vi "Strategy 5_Autotuning PID_With GUI Modified for Testing_Corrupted.vi"() -> ()   [LabVIEW 2018]
doc: "This example demonstrates how to use the PID Design function to obtain PID parameters based on measured process."
uses:
  <vilib>/DAQmx/write.llb/DAQmx Write (Digital 1D Bool 1Chan 1Samp).vi
  <vilib>/DAQmx/read.llb/DAQmx Read (Analog 1D DBL NChan 1Samp).vi
  <vilib>/Instr/_visa.llb/VISA Configure Serial Port (Instr).vi
  <vilib>/DAQmx/create/channels.llb/DAQmx Create Channel (DO-Digital Output).vi
  <vilib>/DAQmx/miscellaneous.llb/DAQmx Fill In Error Info.vi
  <vilib>/addons/control/pid/pid.llb/PID Advanced (DBL).vi
  <vilib>/addons/control/pid/autopid.llb/PID Autotuning Design (Ziegler-Nichols).vi
  <vilib>/addons/control/pid/autopid.llb/PID Autotuning Design (Cohen-Coon).vi
  <vilib>/addons/control/pid/autopid.llb/PID Autotuning Design (Chien-Hrones-Reswick).vi
  <vilib>/addons/control/pid/autopid.llb/PID Autotuning Design (Internal Model Control).vi
  <vilib>/addons/control/pid/NI_PID_autopid.lvlib
  <vilib>/addons/control/pid/NI_PID_pid.lvlib
  <vilib>/ptbypt/NI_PtbyPt.lvlib
panel:
  out "Tracker 4 - X,Y,Z":cluster{"x":sgl, "y":sgl, "z":sgl}(graph)
  out "Tracker 3 - X,Y,Z":cluster{"x":sgl, "y":sgl, "z":sgl}(graph)
  out "Tracker 2 - X,Y,Z":cluster{"x":sgl, "y":sgl, "z":sgl}(graph)
  out "Tracker 1 - X,Y,Z":cluster{"x":sgl, "y":sgl, "z":sgl}(graph)
  in  "Set Point 1,5":dbl
  out "Real time Data 1,5":dbl[][](graph)
  in  "Set Point 3,4":dbl
  out "Real time Data 3,4":dbl[][](graph)
  in  "Set Point 2":dbl
  out "Real time Data 2":dbl[][](graph)
  in  "Set Point 7":dbl
  out "Real time Data 7":dbl[][](graph)
  in  "Set Point  6,8,9,10":dbl
  out "Real time Data 6,8,9,10":dbl[][](graph)
  in  "Set Point 11,12":dbl
  out "Real time Data -11,12":dbl[][](graph)
  out "error out":errorcluster {"code" format="%.0x"}
  in  "XYZAER":T1(array[cluster]) {"r" format="%1_6f"; "e" format="%1_6f"; "a" format="%1_6f"; "z" format="%1_6f"; "y" format="%1_6f"; "x" format="%1_6f"}
  out "Start Time Text":string
  out "Stop Time Text":string
  out "Elapsed Time Text":string
  out "HostFrameCount":u32
  out "Loop Iter":i32
  out "PnoData":bool
  in  "stop":bool
  out "?":bool
  in  "Muscle Control":T2(tab)=enum."M-11,12"
  out "Tuned PID gains 12":T3={"proportional gain (Kc)"=1.9838195929127882, "integral time (Ti, min)"=0.01995856284686879, "derivative time (Td, min)"=0.0} {"derivative time (Td, min)" format="%#.6g"; "integral time (Ti, min)" format="%#.6g"; "proportional gain (Kc)" format="%#.6g"}
  in  "Accept gain 12":bool
  in  "Control 12":T4(tab)
  in  "Ziegler-Nichols speed 12":u16(ring) items=["Fast", "Normal", "Slow"]
  in  "Tuning specifications 12":u16(ring) items=["Regulator - 0 %", "Regulator -  20%", "Servo - 0%", "Servo - 20%"]
  in  "Multiplicative factor 12":dbl(slide)=1.0 scale=0.01..100.0
  in  "Type of controller 12":u16(ring)=2 items=["P", "PI", "PID"]
  in  "Stop 12":bool
  in  "PID Gains 12":T3={"proportional gain (Kc)"=0.1625, "integral time (Ti, min)"=1.25, "derivative time (Td, min)"=0.0} {"derivative time (Td, min)" format="%#.6g"; "integral time (Ti, min)" format="%#.6g"; "proportional gain (Kc)" format="%#.6g"}
  in  "Autotune 12":bool
  in  "Reinitialize 12":bool
  in  "Excitation 12":dbl=0.5 format="%.2f"
  in  "Automatic 12":bool=TRUE
  in  "MV: 12":dbl(slide)=20.39115328927357 scale=-100.0..100.0
  out "PWM Output 12":bool
  in  "Median sample length 21":i32=100
  in  "INLET 1,5 ON/OFF 3":bool=TRUE
  out "Tuned PID gains 9":T3={"proportional gain (Kc)"=1.9838195929127882, "integral time (Ti, min)"=0.01995856284686879, "derivative time (Td, min)"=0.0} {"derivative time (Td, min)" format="%#.6g"; "integral time (Ti, min)" format="%#.6g"; "proportional gain (Kc)" format="%#.6g"}
  in  "Accept gain 9":bool
  in  "Type of controller 9":u16(ring)=2 items=["P", "PI", "PID"]
  in  "Excitation 9":dbl=0.5 format="%.2f"
  in  "Control 9":T4(tab)
  in  "Ziegler-Nichols speed 9":u16(ring) items=["Fast", "Normal", "Slow"]
  in  "Tuning specifications 9":u16(ring) items=["Regulator - 0 %", "Regulator -  20%", "Servo - 0%", "Servo - 20%"]
  in  "Multiplicative factor 9":dbl(slide)=1.0 scale=0.01..100.0
  in  "Stop 9":bool
  in  "PID Gains 9":T3={"proportional gain (Kc)"=0.1625, "integral time (Ti, min)"=1.25, "derivative time (Td, min)"=0.0} {"derivative time (Td, min)" format="%#.6g"; "integral time (Ti, min)" format="%#.6g"; "proportional gain (Kc)" format="%#.6g"}
  in  "Autotune 9":bool
  in  "Reinitialize 9":bool
  in  "Automatic 9":bool=TRUE
  in  "MV: 9":dbl(slide)=20.39115328927357 scale=-100.0..100.0
  out "PWM Output 9":bool
  in  "Median sample length 18":i32=100
  in  "INLET 3,4 ON/OFF 2":bool=TRUE
  out "Tuned PID gains 8":T3={"proportional gain (Kc)"=1.9838195929127882, "integral time (Ti, min)"=0.01995856284686879, "derivative time (Td, min)"=0.0} {"derivative time (Td, min)" format="%#.6g"; "integral time (Ti, min)" format="%#.6g"; "proportional gain (Kc)" format="%#.6g"}
  in  "Accept gain 8":bool
  in  "Control 8":T4(tab)
  in  "Ziegler-Nichols speed 8":u16(ring) items=["Fast", "Normal", "Slow"]
  in  "Tuning specifications 8":u16(ring) items=["Regulator - 0 %", "Regulator -  20%", "Servo - 0%", "Servo - 20%"]
  in  "Multiplicative factor 8":dbl(slide)=1.0 scale=0.01..100.0
  in  "Type of controller 8":u16(ring)=2 items=["P", "PI", "PID"]
  in  "Stop 8":bool
  in  "PID Gains 8":T3={"proportional gain (Kc)"=0.1625, "integral time (Ti, min)"=1.25, "derivative time (Td, min)"=0.0} {"derivative time (Td, min)" format="%#.6g"; "integral time (Ti, min)" format="%#.6g"; "proportional gain (Kc)" format="%#.6g"}
  in  "Autotune 8":bool
  in  "Reinitialize 8":bool
  in  "Excitation 8":dbl=0.5 format="%.2f"
  in  "Automatic 8":bool=TRUE
  in  "MV: 8":dbl(slide)=20.39115328927357 scale=-100.0..100.0
  out "PWM Output 8":bool
  in  "Median sample length 17":i32=100
  in  "INLET 2 ON/OFF 2":bool=TRUE
  out "Tuned PID gains 7":T3={"proportional gain (Kc)"=1.9838195929127882, "integral time (Ti, min)"=0.01995856284686879, "derivative time (Td, min)"=0.0} {"derivative time (Td, min)" format="%#.6g"; "integral time (Ti, min)" format="%#.6g"; "proportional gain (Kc)" format="%#.6g"}
  in  "Accept gain 7":bool
  in  "Control 7":T4(tab)
  in  "Ziegler-Nichols speed 7":u16(ring) items=["Fast", "Normal", "Slow"]
  in  "Tuning specifications 7":u16(ring) items=["Regulator - 0 %", "Regulator -  20%", "Servo - 0%", "Servo - 20%"]
  in  "Multiplicative factor 7":dbl(slide)=1.0 scale=0.01..100.0
  in  "Type of controller 7":u16(ring)=2 items=["P", "PI", "PID"]
  in  "Stop 7":bool
  in  "PID Gains 7":T3={"proportional gain (Kc)"=0.1625, "integral time (Ti, min)"=1.25, "derivative time (Td, min)"=0.0} {"derivative time (Td, min)" format="%#.6g"; "integral time (Ti, min)" format="%#.6g"; "proportional gain (Kc)" format="%#.6g"}
  in  "Autotune 7":bool
  in  "Reinitialize 7":bool
  in  "Excitation 7":dbl=0.5 format="%.2f"
  in  "Automatic 7":bool=TRUE
  in  "MV: 7":dbl(slide)=20.39115328927357 scale=-100.0..100.0
  out "PWM Output 7":bool
  in  "Median sample length 16":i32=100
  in  "INLET 7 ON/OFF 2":bool=TRUE
  out "Tuned PID gains 6":T3={"proportional gain (Kc)"=1.9838195929127882, "integral time (Ti, min)"=0.01995856284686879, "derivative time (Td, min)"=0.0} {"derivative time (Td, min)" format="%#.6g"; "integral time (Ti, min)" format="%#.6g"; "proportional gain (Kc)" format="%#.6g"}
  in  "Accept gain 6":bool
  in  "Control 6":T4(tab)
  in  "Ziegler-Nichols speed 6":u16(ring) items=["Fast", "Normal", "Slow"]
  in  "Tuning specifications 6":u16(ring) items=["Regulator - 0 %", "Regulator -  20%", "Servo - 0%", "Servo - 20%"]
  in  "Multiplicative factor 6":dbl(slide)=1.0 scale=0.01..100.0
  in  "Type of controller 6":u16(ring)=2 items=["P", "PI", "PID"]
  in  "Stop 6":bool
  in  "PID Gains 6":T3={"proportional gain (Kc)"=0.1625, "integral time (Ti, min)"=1.25, "derivative time (Td, min)"=0.0} {"derivative time (Td, min)" format="%#.6g"; "integral time (Ti, min)" format="%#.6g"; "proportional gain (Kc)" format="%#.6g"}
  in  "Autotune 6":bool
  in  "Reinitialize 6":bool
  in  "Excitation 6":dbl=0.5 format="%.2f"
  in  "Automatic 6":bool=TRUE
  in  "MV: 6":dbl(slide)=20.39115328927357 scale=-100.0..100.0
  out "PWM Output 6":bool
  in  "Median sample length 15":i32=100
  in  "INLET 6 ON/OFF 2":bool=TRUE
  in  "INLET":bool=TRUE
  out "PWM Output":bool
  in  "MV:":dbl(slide)=20.39115328927357 scale=-100.0..100.0
  in  "Median sample length":i32=100
  in  "Excitation":dbl=0.5 format="%.2f"
  in  "Type of controller":u16(ring)=2 items=["P", "PI", "PID"]
  in  "Control":T4(tab)
  in  "Ziegler-Nichols speed":u16(ring) items=["Fast", "Normal", "Slow"]
  in  "Tuning specifications":u16(ring) items=["Regulator - 0 %", "Regulator -  20%", "Servo - 0%", "Servo - 20%"]
  in  "Multiplicative factor":dbl(slide)=1.0 scale=0.01..100.0
  in  "Automatic":bool=TRUE
  in  "Reinitialize":bool
  in  "Accept gain":bool
  out "Tuned PID gains":T3={"proportional gain (Kc)"=1.9838195929127882, "integral time (Ti, min)"=0.01995856284686879, "derivative time (Td, min)"=0.0} {"derivative time (Td, min)" format="%#.6g"; "integral time (Ti, min)" format="%#.6g"; "proportional gain (Kc)" format="%#.6g"}
  in  "Autotune":bool
  in  "PID Gains":T3={"proportional gain (Kc)"=0.1625, "integral time (Ti, min)"=1.25, "derivative time (Td, min)"=0.0} {"derivative time (Td, min)" format="%#.6g"; "integral time (Ti, min)" format="%#.6g"; "proportional gain (Kc)" format="%#.6g"}
  in  "Stop":bool
  in  "M-11,12":i32=5
  in  "M-6,8,9,10":i32=5
  in  "M-7":i32=5
  in  "M-2":i32=5
  in  "M-3,4":i32=5
  in  "M-1,5":i32=5
  out "Stimulus operating point 12":dbl=20.314221540357543
  out "Response operating point 12":dbl=51.08345461694337
  out "Identified Plant Parameters 12":T5={"Plant Gain (K)"=1.7609511324977591, "Time Constant (T)"=1.9621978490901302, "Dead Time (L)"=0.22467425343567116}
  out "Control Output 12":dbl[](graph)
  out "Measurement 12":dbl[](graph)
  out "Stimulus operating point 9":dbl=20.314221540357543
  out "Response operating point 9":dbl=51.08345461694337
  out "Identified Plant Parameters 9":T5={"Plant Gain (K)"=1.7609511324977591, "Time Constant (T)"=1.9621978490901302, "Dead Time (L)"=0.22467425343567116}
  out "Control Output 9":dbl[](graph)
  out "Measurement 9":dbl[](graph)
  out "Identified Plant Parameters":T5={"Plant Gain (K)"=1.7609511324977591, "Time Constant (T)"=1.9621978490901302, "Dead Time (L)"=0.22467425343567116}
  out "Control Output":dbl[](graph)
  out "Measurement":dbl[](graph)
  out "Stimulus operating point":dbl=20.314221540357543
  out "Response operating point":dbl=51.08345461694337
  out "Stimulus operating point 6":dbl=20.314221540357543
  out "Response operating point 6":dbl=51.08345461694337
  out "Identified Plant Parameters 6":T5={"Plant Gain (K)"=1.7609511324977591, "Time Constant (T)"=1.9621978490901302, "Dead Time (L)"=0.22467425343567116}
  out "Control Output 6":dbl[](graph)
  out "Measurement 6":dbl[](graph)
  out "Stimulus operating point 7":dbl=20.314221540357543
  out "Response operating point 7":dbl=51.08345461694337
  out "Identified Plant Parameters 7":T5={"Plant Gain (K)"=1.7609511324977591, "Time Constant (T)"=1.9621978490901302, "Dead Time (L)"=0.22467425343567116}
  out "Control Output 7":dbl[](graph)
  out "Measurement 7":dbl[](graph)
  out "Stimulus operating point 8":dbl=20.314221540357543
  out "Response operating point 8":dbl=51.08345461694337
  out "Identified Plant Parameters 8":T5={"Plant Gain (K)"=1.7609511324977591, "Time Constant (T)"=1.9621978490901302, "Dead Time (L)"=0.22467425343567116}
  out "Control Output 8":dbl[](graph)
  out "Measurement 8":dbl[](graph)
  out "Connected":bool
  out "Running":bool
  out "Position Sensor Data":cluster{dbl, "x":sgl}[](graph)
  out "Sensor Raw Value 2":i32
  in  "COM Port-Sensor 2":refnum<visa-resource-name>="COM5"
  in  "upper/lower infle":enum32{"Page 1", "Page 2"}(tab)
  out "Force in Kilograms":dbl(graph)
  out "Force in Newtons":dbl(graph)
  in  "lower/upper infle":enum32{"Page 1", "Page 2"}(tab)
  out "Force in Newtons 2":dbl(graph)
  out "Force in Kilograms 2":dbl(graph)
  in  "COM Port-Sensor 1":refnum<visa-resource-name>="COM4"
  out "Sensor Raw Value":i32
  in  "Tab Control":T6(tab)
  in  "Instructions":string="Overview: This example demonstrates how to use the PID Autotuning Design to obtain PID parameters based on setpoint and process variable collected in another loop.\nInstructions:\n1. Run the VI and wait until the process variable (PV) reaches near setpoint (SP).\n2.  In the PID Autotuning Design section, select the type of algorithm, type of controller and excitation amplitude for the 'open loop step response'. Then, click Autotune to start the process. Select the Identified Plant Parameter tab and see the results from the identification.\n3.  When the tuned PID gains do not change anymore, the identification is done and you have the option to accept by clicking Accept gain, which will transfer the new gain to PID Gains.\n4. Click the Autotune button again to go back to the automatic control state. You can try different options and repeat this process.\n5. Click Stop to stop the VI.\n"
  # "Pressure Alarm"
  # "Force Sensor Data"
  # "Position Sensor Data"
  # "PID Controller"
  # "PID Autotuning Design"
  # "No additional parameters"
  # "PID Controller"
  # "PID Autotuning Design"
  # "No additional parameters"
  # "PID Controller"
  # "PID Autotuning Design"
  # "No additional parameters"
  # "PID Controller"
  # "PID Autotuning Design"
  # "No additional parameters"
  # "PID Controller"
  # "PID Autotuning Design"
  # "No additional parameters"
  # "Muscle Control"
  # "PID Controller"
  # "PID Autotuning Design"
  # "No additional parameters"
  # "Pressure Cut Off to trigger the alarm"
  # "M-11,12"
  # "M-3,4"
  # "M-1,5"
  # "M-6,8,9,10"
  # "M-7"
  # "M-2"
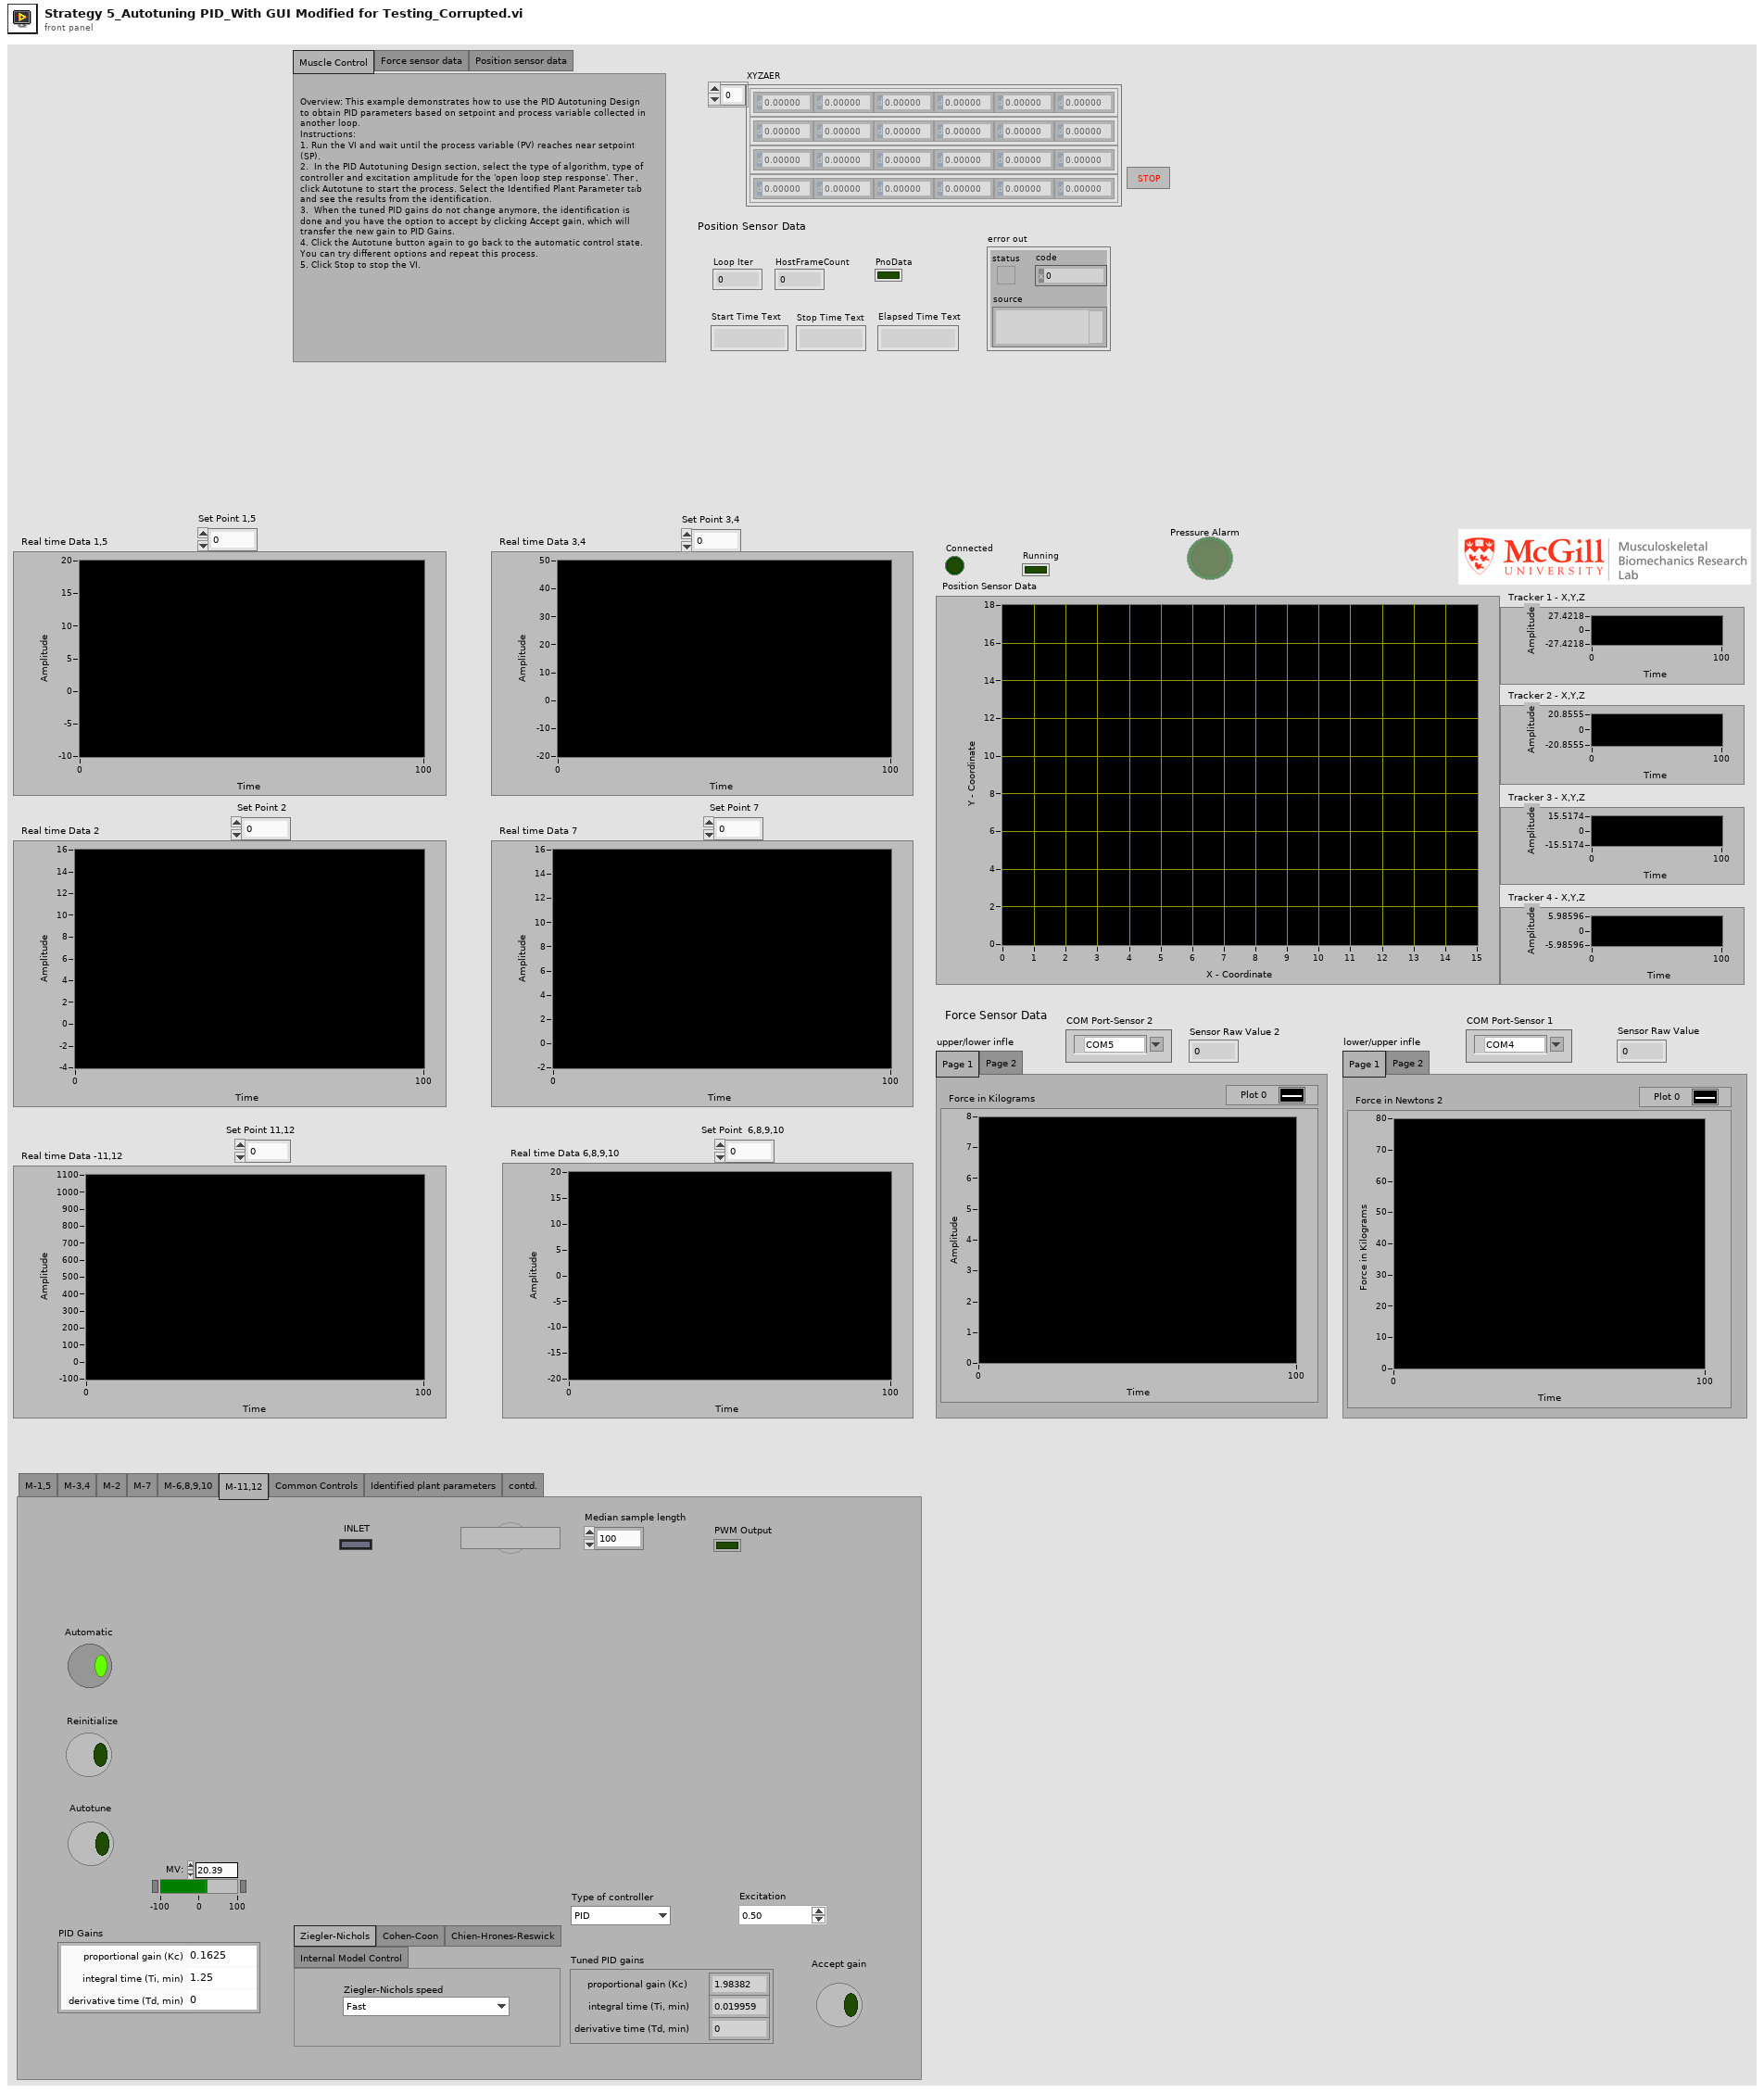
[diagram p1: front panel]
types:
  T1 = cluster{"x":sgl, "y":sgl, "z":sgl, "a":sgl, "e":sgl, "r":sgl}[]
  T2 = enum32{"M-1,5", "M-3,4", "M-2", "M-7", "M-6,8,9,10", "M-11,12", "Common Controls", "Identified plant parameters", "contd."}
  T3 = cluster{"proportional gain (Kc)":dbl, "integral time (Ti, min)":dbl, "derivative time (Td, min)":dbl}
  T4 = enum32{"Ziegler-Nichols", "Cohen-Coon", "Chien-Hrones-Reswick", "Internal Model Control"}
  T5 = cluster{"Plant Gain (K)":dbl, "Time Constant (T)":dbl, "Dead Time (L)":dbl}
  T6 = enum32{"Muscle Control", "Force sensor data", "Position sensor data"}
  T7 = cluster{"static gain":dbl, "lag (s)":dbl, "deadtime (s)":dbl, "load":dbl, "deadband":dbl, "sensor noise":dbl, "initial PV":dbl, "plant noise":dbl}
  T8 = cluster{"x":sgl, "y":sgl, "z":sgl, "a":sgl, "e":sgl, "r":sgl}
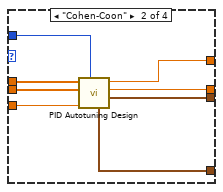
[diagram p2: hidden frame]
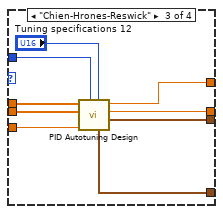
[diagram p3: hidden frame]
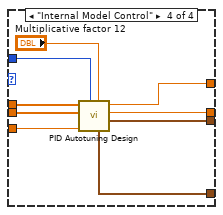
[diagram p4: hidden frame]
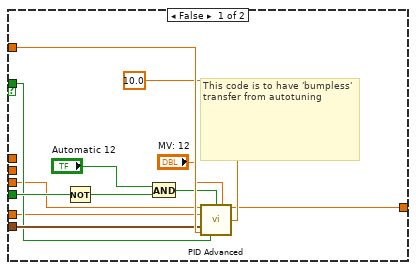
[diagram p6: hidden frame]
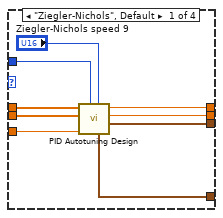
[diagram p7: hidden frame]
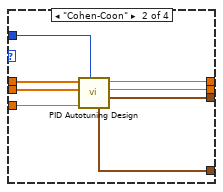
[diagram p8: hidden frame]
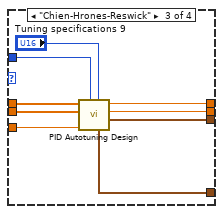
[diagram p9: hidden frame]
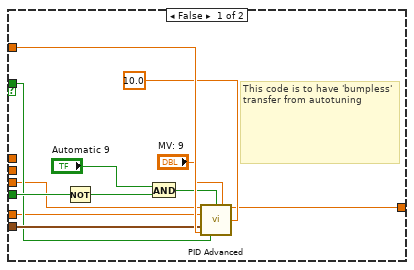
[diagram p11: hidden frame]
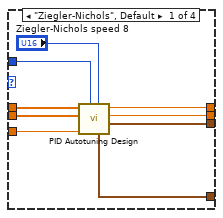
[diagram p12: hidden frame]
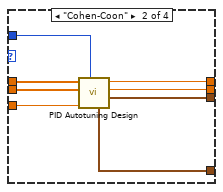
[diagram p13: hidden frame]
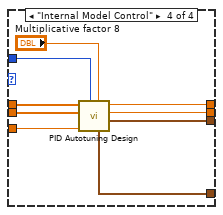
[diagram p14: hidden frame]
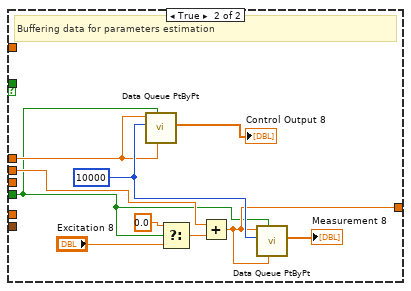
[diagram p16: hidden frame]
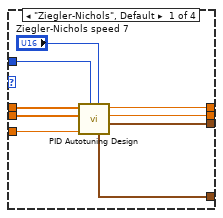
[diagram p17: hidden frame]
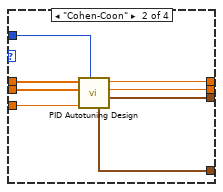
[diagram p18: hidden frame]
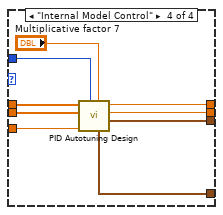
[diagram p19: hidden frame]
diagram:
  w19 = 0.0 ("output")
  w22 = FALSE ("Stop")
  w25 = 0.0 ("output")
  w28 = FALSE ("Stop")
  w31 = 0.0 ("output")
  w34 = FALSE ("Stop")
  w36 = 0.0 ("output")
  w42 = 0.0 ("output")
  w45 = FALSE ("Stop")
  w50 = 2400  # BufferFrameCount
  w83 = 0.0 ("output")
  # "Muscle-1,5 PID CONTROL LOOP (Auto Tuning)"
  # "Muscle-3,4 PID CONTROL LOOP (Auto Tuning)"
  # "Muscle-2 PID CONTROL LOOP (Auto Tuning)"
  # "Muscle-7 PID CONTROL LOOP (Auto Tuning)"
  # "Muscle-6,8,9,10 PID CONTROL LOOP (Auto Tuning)"
  # "Muscle-11,12 PID CONTROL LOOP (Auto Tuning)"
  # "FORCE SENSOR CONTROL LOOP"
  # "POSITION SENSOR CONTROL LOOP"
  # "Pressure Alarm"
  # "8. Close Tracker connection."
  # "3. Query Max num sensors supported by the tracker."
  # "4. Allocate raw buffer to hold 2400 frames of data."
  # "5. Start Continuous mode."
  # "7. Stop Continuous mode."
  # "6. Start the loop. Loop exits when Stop Button is hit."
  n1 = Obtain Queue(element data type=0.0) -> (queue out=w12:refnum<queue>)  [unwired: 4 in, 2 out]
  n2 = while {
    shift-left: 0.0 ("Plant Output") -> [w202]
    shift-right: [w197] -> _
    tunnel: w45 -> [_]
    shift-right: [w183] -> _
    shift-left: 0.01 -> [w181]
    shift-right: [w156] -> _
    shift-left: TRUE -> [w180]
    shift-right: [w158] -> _
    shift-left: w42 -> [w179]
    shift-right: [w182] -> _
    shift-left: w42 -> [w178]
    tunnel: [w153] -> w41
    tunnel: [w140] -> w2
    tunnel: w12 -> [w138]
    stop <- "Stop 6" stop-if-true
    w91 = 1 items=["one channel for each line", "one channel for all lines"] ("line grouping")
    w99 = 1 items=["one channel for each line", "one channel for all lines"] ("line grouping")
    w107 = 1 items=["one channel for each line", "one channel for all lines"] ("line grouping")
    w115 = 1 items=["one channel for each line", "one channel for all lines"] ("line grouping")
    w123 = 1 items=["one channel for each line", "one channel for all lines"] ("line grouping")
    w131 = 1 items=["one channel for each line", "one channel for all lines"] ("line grouping")
    w144 = 1 items=["one channel for each line", "one channel for all lines"] ("line grouping")
    w153 = 0.05 ("Sampling Time dt (s)")
    w161 = 1 items=["one channel for each line", "one channel for all lines"] ("line grouping")
    w169 = 0.5 ("x")
    w196 = T7 {"static gain"=2.5, "lag (s)"=2.5, "deadtime (s)"=0.01, "load"=0.0, "deadband"=0.0, "sensor noise"=0.0, "initial PV"=30.0, "plant noise"=0.0}  # Process parameters
    w198 = FALSE  # Integrator ?
    # "Inlet 11"
    # "Exhaust 10"
    # "Inlet 11"
    # "Exhaust 9"
    # "Inlet 11"
    # "Exhaust 8"
    # "C."
    # "Inlet 11"
    # "Exhaust 6"
    # "B."
    # "A."
    # "A.Output to PWM Logic \nB. Simulated Plant\nC. Draw Chart"
    # "Main PID Loop Control"
    n3 = Dequeue Element(queue=w138) -> (element=w139:dbl)  [unwired: 2 in, 3 out]
    n4 = Multiply(x=w153, y=1000.0) -> (x*y=w195:dbl)
    n5 = Not(x="Autotune 6") -> (.not. x?=w199:bool)
    n6 = feedback #1() -> (w204:bool)  [unwired: 1 in]
    n7 = feedback-in #1("Autotune 6") -> ()
    n8 = Wait Until Next ms Multiple(millisecond multiple=w195) -> ()  [unwired: 1 out]
    n9 = Exclusive Or(1:w204, 2:"Autotune 6") -> (0:w203:bool)
    n10 = feedback #2() -> (w201:dbl)  [unwired: 1 in]
    n11 = Multiply(x=w139, y=-1000.0) -> (x*y=w185:dbl)
    n12 = call <vilib>:"Median PtByPt.vi"("sample length"="Median sample length 15", "x"=w185) -> ("median"=w184:dbl)  [unwired: 2 in, 1 out]
    n13 = Square(x=w184) -> (x^2=w192:dbl)
    n14 = Multiply(x=w184, y=16.572) -> (x*y=w188:dbl)
    n15 = Multiply(x=w192, y=-0.06) -> (x*y=w189:dbl)
    n16 = Add(x=w188, y=w189) -> (x+y=w187:dbl)
    n17 = Add(x=-1011.3, y=w187) -> (x+y=w151:dbl)
    n18 = case shown="False" "Autotune 6" {
      tunnel: w153 -> [w219 _]
      tunnel: [w208 w224] -> w158
      tunnel: w202 -> [_ w223]
      tunnel: "PID Gains 6" -> [w218 _]
      tunnel: "Reinitialize 6" -> [w215 _]
      tunnel: w203 -> [w217 w222]
      tunnel: w201 -> [_ w226]
      tunnel: w151 -> [w211 _]
      tunnel: "Set Point  6,8,9,10" -> [w210 _]
      frame False {
        # "This code is to have 'bumpless' transfer from autotuning"
        n19 = Not(x=w217) -> (.not. x?=w214:bool)
        n20 = And(x="Automatic 6", y=w214) -> (x .and. y?=w216:bool)
        n21 = call-poly <vilib>:"PID Advanced.vi"("setpoint"=w210, "auto? (T)"=w216, "manual control"="MV: 6", "process variable"=w211, "alpha"=10.0, "PID gains"=w218, "dt (s)"=w219, "reinitialize? (F)"=w215) -> ("output"=w208:dbl)  [unwired: 6 in, 1 out]
      }
      frame True {
        w229 = 10000 ("sample length")
        # "Buffering data for parameters estimation"
        n22 = call <vilib>:"Data Queue PtByPt.vi"("initial queue element"=w223, "initialize"=w222, "sample length"=w229, "input data point"=w223) -> ("Current Queue"=→"Control Output 6":dbl[])  [unwired: 3 in, 4 out]
        n23 = Select(t=0.0, s=w222, f="Excitation 6") -> (s? t:f=w227:dbl)
        n24 = Add(x=w226, y=w227) -> (x+y=w224:dbl)
        n25 = call <vilib>:"Data Queue PtByPt.vi"("initial queue element"=w224, "initialize"=w222, "sample length"=w229, "input data point"=w224) -> ("Current Queue"=→"Measurement 6":dbl[])  [unwired: 3 in, 4 out]
      }
    }
    n26 = feedback-in #2(w158, w199) -> ()
    n27 = Greater?(x=w151, y="M-6,8,9,10") -> (0:w140:bool)
    n28 = Add(x=w181, y=w169) -> (x+y=w170:dbl)
    n29 = Subtract(x=w181, y=w169) -> (x-y=w168:dbl)
    n30 = Equal?(x=w179, y=w158) -> (x = y?=w176:bool)
    n31 = Greater?(x=w158, y=w179) -> (0:w175:bool)
    n32 = Select(t=w180, s=w176, f=w175) -> (s? t:f=w156:bool)
    "PWM Output 6" <- w156
    n33 = call "Plant System.vi"("Integrator ?"=w198, "Plant Input"=w158, "dt (s)"=w153, "process parameters"=w196) -> ("Plant Output"=w197:dbl)  [unwired: 11 in]
    n34 = Increment(x="Set Point  6,8,9,10") -> (x+1=w174:dbl)
    n35 = Decrement(x="Set Point  6,8,9,10") -> (x-1=w173:dbl)
    n36 = Select(t=w170, s=w156, f=w168) -> (s? t:f=w183:dbl)
    n37 = call-poly <vilib>:"DAQmx Create Virtual Channel.vi"("lines"=tag "cDAQ1Mod1/port0/line3", "line grouping"=w115) -> ("task out"=w117:refnum<k21>, "error out"=w116:errorcluster)  [unwired: 12 in]
    n38 = call-poly <vilib>:"DAQmx Create Virtual Channel.vi"("lines"=tag "cDAQ1Mod2/port0/line3", "line grouping"=w107) -> ("task out"=w109:refnum<k21>, "error out"=w108:errorcluster)  [unwired: 12 in]
    n39 = Select(t=w174, s=w156, f=w173) -> (s? t:f=w172:dbl)
    n40 = Not(x=w156) -> (.not. x?=w155:bool)
    n41 = call-poly <vilib>:"DAQmx Create Virtual Channel.vi"("lines"=tag "cDAQ1Mod1/port0/line4", "line grouping"=w161) -> ("task out"=w163:refnum<k21>, "error out"=w162:errorcluster)  [unwired: 12 in]
    n42 = call-poly <vilib>:"DAQmx Create Virtual Channel.vi"("lines"=tag "cDAQ1Mod2/port0/line4", "line grouping"=w144) -> ("task out"=w146:refnum<k21>, "error out"=w145:errorcluster)  [unwired: 12 in]
    n43 = Build Array(w151, "Set Point  6,8,9,10", w172) -> (w171:dbl[])
    n44 = Initialize Array("INLET 6 ON/OFF 2", 1 ("dimension size")) -> (w88:bool[])
    n45 = Initialize Array(w155, 1 ("dimension size")) -> (w89:bool[])
    n46 = local write "MV: 6"(w158) -> ()
    n47 = Add(x=w178, y=w181) -> (x+y=w182:dbl)
    n48 = Build Array(w171) -> (→"Real time Data 6,8,9,10":dbl[][])
    n49 = call-poly <vilib>:"DAQmx Write.vi"("task/channels in"=w117, "auto start"=TRUE, "data"=w89, "error in"=w116) -> ("task out"=w119:refnum<k21>, "error out"=w120:errorcluster)  [unwired: 9 in, 1 out]
    n50 = call-poly <vilib>:"DAQmx Write.vi"("task/channels in"=w109, "auto start"=TRUE, "data"=w88, "error in"=w108) -> ("task out"=w111:refnum<k21>, "error out"=w112:errorcluster)  [unwired: 9 in, 1 out]
    n51 = call-poly <vilib>:"DAQmx Write.vi"("task/channels in"=w163, "auto start"=TRUE, "data"=w89, "error in"=w162) -> ("task out"=w165:refnum<k21>, "error out"=w166:errorcluster)  [unwired: 9 in, 1 out]
    n52 = call-poly <vilib>:"DAQmx Write.vi"("task/channels in"=w146, "auto start"=TRUE, "data"=w88, "error in"=w145) -> ("task out"=w148:refnum<k21>, "error out"=w149:errorcluster)  [unwired: 9 in, 1 out]
    n53 = call <vilib>:"DAQmx Clear Task.vi"("task in"=w119, "error in"=w120) -> ("error out"=w114:errorcluster)  [unwired: 13 in]
    n54 = call <vilib>:"DAQmx Clear Task.vi"("task in"=w111, "error in"=w112) -> ("error out"=w106:errorcluster)  [unwired: 13 in]
    n55 = call <vilib>:"DAQmx Clear Task.vi"("task in"=w165, "error in"=w166) -> ("error out"=w160:errorcluster)  [unwired: 13 in]
    n56 = call <vilib>:"DAQmx Clear Task.vi"("task in"=w148, "error in"=w149) -> ("error out"=w143:errorcluster)  [unwired: 13 in]
    n57 = call <vilib>:"Simple Error Handler.vi"("error in (no error)"=w114) -> ()  [unwired: 4 in, 5 out]
    n58 = call <vilib>:"Simple Error Handler.vi"("error in (no error)"=w106) -> ()  [unwired: 4 in, 5 out]
    n59 = call <vilib>:"Simple Error Handler.vi"("error in (no error)"=w160) -> ()  [unwired: 4 in, 5 out]
    n60 = call <vilib>:"Simple Error Handler.vi"("error in (no error)"=w143) -> ()  [unwired: 4 in, 5 out]
    n61 = call-poly <vilib>:"DAQmx Create Virtual Channel.vi"("lines"=tag "cDAQ1Mod8/port0/line6", "line grouping"=w99) -> ("task out"=w101:refnum<k21>, "error out"=w100:errorcluster)  [unwired: 12 in]
    n62 = call-poly <vilib>:"DAQmx Create Virtual Channel.vi"("lines"=tag "cDAQ1Mod7/port0/line5", "line grouping"=w91) -> ("task out"=w93:refnum<k21>, "error out"=w92:errorcluster)  [unwired: 12 in]
    n63 = call-poly <vilib>:"DAQmx Create Virtual Channel.vi"("lines"=tag "cDAQ1Mod8/port0/line3", "line grouping"=w131) -> ("task out"=w133:refnum<k21>, "error out"=w132:errorcluster)  [unwired: 12 in]
    n64 = call-poly <vilib>:"DAQmx Create Virtual Channel.vi"("lines"=tag "cDAQ1Mod7/port0/line2", "line grouping"=w123) -> ("task out"=w125:refnum<k21>, "error out"=w124:errorcluster)  [unwired: 12 in]
    n65 = call-poly <vilib>:"DAQmx Write.vi"("task/channels in"=w101, "auto start"=TRUE, "data"=w89, "error in"=w100) -> ("task out"=w103:refnum<k21>, "error out"=w104:errorcluster)  [unwired: 9 in, 1 out]
    n66 = call-poly <vilib>:"DAQmx Write.vi"("task/channels in"=w93, "auto start"=TRUE, "data"=w88, "error in"=w92) -> ("task out"=w95:refnum<k21>, "error out"=w96:errorcluster)  [unwired: 9 in, 1 out]
    n67 = call-poly <vilib>:"DAQmx Write.vi"("task/channels in"=w133, "auto start"=TRUE, "data"=w89, "error in"=w132) -> ("task out"=w135:refnum<k21>, "error out"=w136:errorcluster)  [unwired: 9 in, 1 out]
    n68 = call-poly <vilib>:"DAQmx Write.vi"("task/channels in"=w125, "auto start"=TRUE, "data"=w88, "error in"=w124) -> ("task out"=w127:refnum<k21>, "error out"=w128:errorcluster)  [unwired: 9 in, 1 out]
    n69 = call <vilib>:"DAQmx Clear Task.vi"("task in"=w103, "error in"=w104) -> ("error out"=w98:errorcluster)  [unwired: 13 in]
    n70 = call <vilib>:"DAQmx Clear Task.vi"("task in"=w95, "error in"=w96) -> ("error out"=w90:errorcluster)  [unwired: 13 in]
    n71 = call <vilib>:"DAQmx Clear Task.vi"("task in"=w135, "error in"=w136) -> ("error out"=w130:errorcluster)  [unwired: 13 in]
    n72 = call <vilib>:"DAQmx Clear Task.vi"("task in"=w127, "error in"=w128) -> ("error out"=w122:errorcluster)  [unwired: 13 in]
    n73 = call <vilib>:"Simple Error Handler.vi"("error in (no error)"=w98) -> ()  [unwired: 4 in, 5 out]
    n74 = call <vilib>:"Simple Error Handler.vi"("error in (no error)"=w90) -> ()  [unwired: 4 in, 5 out]
    n75 = call <vilib>:"Simple Error Handler.vi"("error in (no error)"=w130) -> ()  [unwired: 4 in, 5 out]
    n76 = call <vilib>:"Simple Error Handler.vi"("error in (no error)"=w122) -> ()  [unwired: 4 in, 5 out]
  }
  n77 = local write "Stop 6"(w45) -> ()
  n78 = while {
    tunnel: w45 -> [_]
    tunnel: w41 -> [_]
    stop <- w245 stop-if-true
    w230 = 0.05 ("Sampling Time dt (s)")
    # "If dT and deadtime have similar values, the identification could evaluate deadtime as zero and this generates proportional gain equal to Inf. This code avoid gain changes in this situations."
    # "Autotuning Loop"
    n79 = local read "Control Output 6"() -> (w247:dbl[])
    n80 = local read "Measurement 6"() -> (w246:dbl[])
    n81 = Multiply(x=w230, y=1000.0) -> (x*y=w232:dbl)
    n82 = Wait Until Next ms Multiple(millisecond multiple=w232) -> ()  [unwired: 1 out]
    n83 = case shown="\"Chien-Hrones-Reswick\"" "Control 6" {
      tunnel: w247 -> [w256 w264 w273 w282]
      tunnel: w246 -> [w255 w263 w272 w281]
      tunnel: [w254 w262 w271 w280] -> w235
      tunnel: [w253 w261 w270 w279] -> w234
      tunnel: w230 -> [w252 w260 w269 w278]
      tunnel: [w251 w259 w268 w277] -> w233
      tunnel: [w250 w258 w267 w276] -> w237
      tunnel: "Type of controller 6" -> [w249 w257 w266 w275]
      frame "Ziegler-Nichols", Default {
        n84 = call-poly <vilib>:"PID Autotuning Design.vi"("Ziegler-Nichols Speed"="Ziegler-Nichols speed 6", "Type of Controller"=w249, "dt (s)"=w252, "Response signal"=w255, "Stimulus signal"=w256) -> ("PID gains"=w250:T3, "response operating point"=w253:dbl, "stimulus operating point"=w254:dbl, "Plant Parameters"=w251:T5)  [unwired: 3 in]
      }
      frame "Cohen-Coon" {
        n85 = call-poly <vilib>:"PID Autotuning Design.vi"("Type of Controller"=w257, "dt (s)"=w260, "Response signal"=w263, "Stimulus signal"=w264) -> ("PID gains"=w258:T3, "response offset"=w261:dbl, "stimulus offset"=w262:dbl, "Plant Parameters"=w259:T5)  [unwired: 4 in]
      }
      frame "Chien-Hrones-Reswick" {
        n86 = call-poly <vilib>:"PID Autotuning Design.vi"("Tuning specifications"="Tuning specifications 6", "Type of Controller"=w266, "dt (s)"=w269, "Response signal"=w272, "Stimulus signal"=w273) -> ("PID gains"=w267:T3, "response offset"=w270:dbl, "stimulus offset"=w271:dbl, "Plant Parameters"=w268:T5)  [unwired: 3 in]
      }
      frame "Internal Model Control" {
        n87 = call-poly <vilib>:"PID Autotuning Design.vi"("Desired Time Constant (tau_c)"="Multiplicative factor 6", "Type of Controller"=w275, "dt (s)"=w278, "Response signal"=w281, "Stimulus signal"=w282) -> ("PID gains"=w276:T3, "response offset"=w279:dbl, "stimulus offset"=w280:dbl, "Plant Parameters"=w277:T5)  [unwired: 3 in]
      }
    }
    "Stimulus operating point 6" <- w235
    "Response operating point 6" <- w234
    "Identified Plant Parameters 6" <- w233
    n88 = Unbundle(w237) -> ("proportional gain (Kc)"=w240:dbl)  [unwired: 2 out]
    n89 = Equal?(x=w240, y=inf) -> (x = y?=w239:bool)
    n90 = feedback #3() -> (w238:T3)  [unwired: 1 in]
    n91 = Select(t=w238, s=w239, f=w237) -> (s? t:f=w236:T3)
    "Tuned PID gains 6" <- w236
    n92 = feedback-in #3(w236) -> ()
    n93 = case shown="True" "Accept gain 6" {
      tunnel: w236 -> [_ w283]
      frame False {
      }
      frame True {
        n94 = local write "PID Gains 6"(w283) -> ()
      }
    }
    n95 = local read "Stop 6"() -> (w245:bool)
  }
  n96 = local write "Stop"(FALSE ("Stop")) -> ()
  n97 = call-poly "VISA Configure Serial Port"("VISA resource name"="COM Port-Sensor 1") -> ("VISA resource name out"=w78:refnum<visa-resource-name>, "error out"=w77:errorcluster)  [unwired: 9 in, 4 out]
  n98 = call-poly "VISA Configure Serial Port"("VISA resource name"="COM Port-Sensor 2") -> ("VISA resource name out"=w73:refnum<visa-resource-name>, "error out"=w72:errorcluster)  [unwired: 9 in, 4 out]
  n99 = while {
    stop <- w299 stop-if-true
    w284 = 0.05 ("Sampling Time dt (s)")
    # "If dT and deadtime have similar values, the identification could evaluate deadtime as zero and this generates proportional gain equal to Inf. This code avoid gain changes in this situations."
    # "Autotuning Loop"
    n100 = local read "Control Output"() -> (w301:dbl[])
    n101 = local read "Measurement"() -> (w300:dbl[])
    n102 = Multiply(x=w284, y=1000.0) -> (x*y=w286:dbl)
    n103 = Wait Until Next ms Multiple(millisecond multiple=w286) -> ()  [unwired: 1 out]
    n104 = case shown="\"Ziegler-Nichols\", Default" "Control" {
      tunnel: w301 -> [w310 w318 w327 w336]
      tunnel: w300 -> [w309 w317 w326 w335]
      tunnel: [w308 w316 w325 w334] -> w289
      tunnel: [w307 w315 w324 w333] -> w288
      tunnel: w284 -> [w306 w314 w323 w332]
      tunnel: [w305 w313 w322 w331] -> w287
      tunnel: [w304 w312 w321 w330] -> w291
      tunnel: "Type of controller" -> [w303 w311 w320 w329]
      frame "Ziegler-Nichols", Default {
        n105 = call-poly <vilib>:"PID Autotuning Design.vi"("Ziegler-Nichols Speed"="Ziegler-Nichols speed", "Type of Controller"=w303, "dt (s)"=w306, "Response signal"=w309, "Stimulus signal"=w310) -> ("PID gains"=w304:T3, "response operating point"=w307:dbl, "stimulus operating point"=w308:dbl, "Plant Parameters"=w305:T5)  [unwired: 3 in]
      }
      frame "Cohen-Coon" {
        n106 = call-poly <vilib>:"PID Autotuning Design.vi"("Type of Controller"=w311, "dt (s)"=w314, "Response signal"=w317, "Stimulus signal"=w318) -> ("PID gains"=w312:T3, "response offset"=w315:dbl, "stimulus offset"=w316:dbl, "Plant Parameters"=w313:T5)  [unwired: 4 in]
      }
      frame "Chien-Hrones-Reswick" {
        n107 = call-poly <vilib>:"PID Autotuning Design.vi"("Tuning specifications"="Tuning specifications", "Type of Controller"=w320, "dt (s)"=w323, "Response signal"=w326, "Stimulus signal"=w327) -> ("PID gains"=w321:T3, "response offset"=w324:dbl, "stimulus offset"=w325:dbl, "Plant Parameters"=w322:T5)  [unwired: 3 in]
      }
      frame "Internal Model Control" {
        n108 = call-poly <vilib>:"PID Autotuning Design.vi"("Desired Time Constant (tau_c)"="Multiplicative factor", "Type of Controller"=w329, "dt (s)"=w332, "Response signal"=w335, "Stimulus signal"=w336) -> ("PID gains"=w330:T3, "response offset"=w333:dbl, "stimulus offset"=w334:dbl, "Plant Parameters"=w331:T5)  [unwired: 3 in]
      }
    }
    "Stimulus operating point" <- w289
    "Response operating point" <- w288
    "Identified Plant Parameters" <- w287
    n109 = Unbundle(w291) -> ("proportional gain (Kc)"=w294:dbl)  [unwired: 2 out]
    n110 = Equal?(x=w294, y=inf) -> (x = y?=w293:bool)
    n111 = feedback #4() -> (w292:T3)  [unwired: 1 in]
    n112 = Select(t=w292, s=w293, f=w291) -> (s? t:f=w290:T3)
    "Tuned PID gains" <- w290
    n113 = feedback-in #4(w290) -> ()
    n114 = case shown="True" "Accept gain" {
      tunnel: w290 -> [_ w337]
      frame False {
      }
      frame True {
        n115 = local write "PID Gains"(w337) -> ()
      }
    }
    n116 = local read "Stop"() -> (w299:bool)
  }
  n117 = while {
    shift-right: [w345] -> w79
    shift-left: w78 -> [w341]
    tunnel: w77 -> [w340]
    tunnel: [w342] -> w80
    stop <- w343 stop-if-true
    # "Serial Read Loop"
    n118 = case shown="True" TRUE {
      tunnel: [w357 w361] -> w345
      tunnel: w341 -> [w359 w361]
      tunnel: [w356 w360] -> w342
      tunnel: w340 -> [w358 w360]
      frame True {
        n119 = VISA Read(VISA resource name=w359, byte count=u32 1000, error in (no error)=w358) -> (VISA resource name out=w357:refnum<visa-resource-name>, read buffer=w354:string, error out=w356:errorcluster)  [unwired: 1 out]
        n120 = Decimal String To Number(string=w354) -> (number=w352:i32)  [unwired: 2 in, 1 out]
        "Sensor Raw Value" <- w352
        n121 = call <vilib>:"Median PtByPt.vi"("sample length"=20, "x"=w352) -> ("median"=w350:dbl)  [unwired: 2 in, 1 out]
        n122 = To Double Precision Float(number=w350) -> (double precision float=w346:dbl)
        n123 = Multiply(x=w346, y=0.0292) -> (x*y=w349:dbl)
        "Force in Kilograms 2" <- w349
        n124 = Multiply(x=w349, y=9.81) -> (x*y=→"Force in Newtons 2":dbl)
      }
      frame False {
      }
    }
    n125 = Wait (ms)(milliseconds to wait=u32 5) -> ()  [unwired: 1 out]
    n126 = Or(x=w342, y=FALSE) -> (x .or. y?=w343:bool)
  }
  n127 = while {
    shift-right: [w369] -> w47
    shift-left: w73 -> [w365]
    tunnel: w72 -> [w364]
    tunnel: [w366] -> w74
    stop <- w367 stop-if-true
    # "Serial Read Loop"
    n128 = case shown="True" TRUE {
      tunnel: [w381 w385] -> w369
      tunnel: w365 -> [w383 w385]
      tunnel: [w380 w384] -> w366
      tunnel: w364 -> [w382 w384]
      frame True {
        n129 = VISA Read(VISA resource name=w383, byte count=u32 1000, error in (no error)=w382) -> (VISA resource name out=w381:refnum<visa-resource-name>, read buffer=w378:string, error out=w380:errorcluster)  [unwired: 1 out]
        n130 = Decimal String To Number(string=w378) -> (number=w374:i32)  [unwired: 2 in, 1 out]
        "Sensor Raw Value 2" <- w374
        n131 = call <vilib>:"Median PtByPt.vi"("sample length"=20, "x"=w374) -> ("median"=w375:dbl)  [unwired: 2 in, 1 out]
        n132 = To Double Precision Float(number=w375) -> (double precision float=w371:dbl)
        n133 = Multiply(x=w371, y=0.0238) -> (x*y=w370:dbl)
        "Force in Kilograms" <- w370
        n134 = Multiply(x=w370, y=9.81) -> (x*y=→"Force in Newtons":dbl)
      }
      frame False {
      }
    }
    n135 = Or(x=w366, y=FALSE) -> (x .or. y?=w367:bool)
    n136 = Wait (ms)(milliseconds to wait=u32 5) -> ()  [unwired: 1 out]
  }
  n137 = VISA Close(VISA resource name=w79, error in (no error)=w80) -> (error out=w81:errorcluster)
  n138 = call <vilib>:"Simple Error Handler.vi"("error in (no error)"=w81) -> ()  [unwired: 1 in, 8 out]
  n139 = VISA Close(VISA resource name=w47, error in (no error)=w74) -> (error out=w75:errorcluster)
  n140 = call <vilib>:"Simple Error Handler.vi"("error in (no error)"=w75) -> ()  [unwired: 1 in, 8 out]
  n141 = stacked-sequence {
    tunnel: [_ w391] -> w54
    tunnel: [_ w390] -> w53
    frame #0 {
      w386 = 0
      w387 = FALSE
      w388 = ""
      # "Initialize Indicators"
      "Connected" <- w387
      "Start Time Text" <- w388
      "Stop Time Text" <- w388
      "Elapsed Time Text" <- w388
      "HostFrameCount" <- w386
      "Running" <- w387
      "Loop Iter" <- w386
      "PnoData" <- w387
    }
    frame #1 {
      # "Connect To Tracker"
      # "2. Initialize Tracker Connection"
      n142 = call <instrlib>:"PDI initialize.vi"() -> ("error out"=w390:errorcluster, "Connected"=w389:bool, "pDev"=w391:u32)  [unwired: 1 in, 4 out]
      n143 = local write "Connected"(w389) -> ()
    }
  }
  n144 = while {
    stop <- FALSE stop-if-true
    # "TRACKER 4"
    # "TRACKER 3"
    # "TRACKER 2"
    # "TRACKER 1"
    n145 = Index Array(array="XYZAER", index #1=0 ("index"), index #2=1 ("index"), index #3=2 ("index"), index #4=3 ("index")) -> (element #1=w424:T8, element #2=w423:T8, element #3=w422:T8, element #4=w421:T8)
    n146 = Unbundle By Name(w424) -> ("x"=w407:sgl, "y"=w406:sgl, "z"=w405:sgl)
    n147 = Unbundle By Name(w423) -> ("x"=w404:sgl, "y"=w403:sgl, "z"=w402:sgl)
    n148 = Multiply(x=w406, y=sgl -1.0) -> (x*y=w415:sgl)
    n149 = Multiply(x=w403, y=-1.0) -> (x*y=w414:dbl)
    n150 = Bundle(w414, "x"=w404) -> (w410:cluster{dbl, "x":sgl})  [unwired: 1 in]
    n151 = Bundle(w415, "x"=w407) -> (w411:cluster{sgl, "x":sgl})  [unwired: 1 in]
    n152 = Unbundle By Name(w422) -> ("x"=w401:sgl, "y"=w400:sgl, "z"=w399:sgl)
    n153 = Unbundle By Name(w421) -> ("x"=w398:sgl, "y"=w397:sgl, "z"=w396:sgl)
    n154 = Multiply(x=w400, y=-1.0) -> (x*y=w413:dbl)
    n155 = Multiply(x=w397, y=-1.0) -> (x*y=w412:dbl)
    n156 = Bundle(w413, "x"=w401) -> (w409:cluster{dbl, "x":sgl})  [unwired: 1 in]
    n157 = Bundle(w412, "x"=w398) -> (w408:cluster{dbl, "x":sgl})  [unwired: 1 in]
    n158 = Build Array(w411, w410, w409, w408) -> (→"Position Sensor Data":cluster{dbl, "x":sgl}[])
    n159 = Bundle("x"=w407, "y"=w406, "z"=w405) -> (→"Tracker 1 - X,Y,Z":cluster{"x":sgl, "y":sgl, "z":sgl})  [unwired: 1 in]
    n160 = Bundle("x"=w404, "y"=w403, "z"=w402) -> (→"Tracker 2 - X,Y,Z":cluster{"x":sgl, "y":sgl, "z":sgl})  [unwired: 1 in]
    n161 = Bundle("x"=w401, "y"=w400, "z"=w399) -> (→"Tracker 3 - X,Y,Z":cluster{"x":sgl, "y":sgl, "z":sgl})  [unwired: 1 in]
    n162 = Bundle("x"=w398, "y"=w397, "z"=w396) -> (→"Tracker 4 - X,Y,Z":cluster{"x":sgl, "y":sgl, "z":sgl})  [unwired: 1 in]
  }
  n163 = call <instrlib>:"PDI util stationcount.vi"("error in (no error)"=w53, "pDev"=w54) -> ("error out"=w52:errorcluster, "dup pDev"=w51:u32, "MaxCount"=w49:i32)  [unwired: 7 out]
  n164 = call <instrlib>:"PDI config setbuffer.vi"("error in (no error)"=w52, "Max sensors"=w49, "FrameCount"=w50, "pDev"=w51) -> ("error out"=w61:errorcluster, "dup pDev"=w62:u32)  [unwired: 6 out]
  n165 = flat-sequence {
    tunnel: w67 -> [_]
    tunnel: [w431] -> w63
    frame #0 {
      # "Get Start Time"
      n166 = Get Date/Time In Seconds() -> (seconds since 1Jan1904=w432:timestamp)
      n167 = Format Date/Time String(seconds (now)=w432) -> (date/time string=w433:string)  [unwired: 2 out]
      n168 = local write "Start Time Text"(w433) -> ()
      n169 = To Double Precision Float(number=w432) -> (double precision float=w431:dbl)
    }
  }
  n170 = call <instrlib>:"PDI action startcont.vi"("error in (no error)"=w61, "pDev"=w62) -> ("error out"=w68:errorcluster, "Running"=w60:bool, "dup pDev"=w67:u32)  [unwired: 7 out]
  n171 = control-ref of="HostFrameCount"() -> (w58:refnum<vi>)
  n172 = local write "Running"(w60) -> ()
  n173 = Obtain Queue(element data type=0.0) -> (queue out=w8:refnum<queue>)  [unwired: 4 in, 2 out]
  n174 = while {
    shift-left: 0.0 ("Plant Output") -> [w516]
    shift-right: [w511] -> _
    tunnel: w28 -> [_]
    shift-right: [w497] -> _
    shift-left: 0.01 -> [w495]
    shift-right: [w470] -> _
    shift-left: TRUE -> [w494]
    shift-right: [w472] -> _
    shift-left: w25 -> [w493]
    shift-right: [w496] -> _
    shift-left: w25 -> [w492]
    tunnel: [w467] -> w24
    tunnel: [w455] -> w16
    tunnel: w8 -> [w453]
    stop <- "Stop 9" stop-if-true
    w438 = 1 items=["one channel for each line", "one channel for all lines"] ("line grouping")
    w446 = 1 items=["one channel for each line", "one channel for all lines"] ("line grouping")
    w458 = 1 items=["one channel for each line", "one channel for all lines"] ("line grouping")
    w467 = 0.05 ("Sampling Time dt (s)")
    w475 = 1 items=["one channel for each line", "one channel for all lines"] ("line grouping")
    w483 = 0.5 ("x")
    w510 = T7 {"static gain"=2.5, "lag (s)"=2.5, "deadtime (s)"=0.01, "load"=0.0, "deadband"=0.0, "sensor noise"=0.0, "initial PV"=30.0, "plant noise"=0.0}  # Process parameters
    w512 = FALSE  # Integrator ?
    # "Inlet 11"
    # "Exhaust 3"
    # "C."
    # "Inlet 11"
    # "Exhaust 4"
    # "B."
    # "A."
    # "A.Output to PWM Logic \nB. Simulated Plant\nC. Draw Chart"
    # "Main PID Loop Control"
    n175 = Dequeue Element(queue=w453) -> (element=w454:dbl)  [unwired: 2 in, 3 out]
    n176 = Multiply(x=w467, y=1000.0) -> (x*y=w509:dbl)
    n177 = Not(x="Autotune 9") -> (.not. x?=w513:bool)
    n178 = feedback #5() -> (w518:bool)  [unwired: 1 in]
    n179 = feedback-in #5("Autotune 9") -> ()
    n180 = Wait Until Next ms Multiple(millisecond multiple=w509) -> ()  [unwired: 1 out]
    n181 = Exclusive Or(1:w518, 2:"Autotune 9") -> (0:w517:bool)
    n182 = feedback #6() -> (w515:dbl)  [unwired: 1 in]
    n183 = Multiply(x=w454, y=-1000.0) -> (x*y=w499:dbl)
    n184 = call <vilib>:"Median PtByPt.vi"("sample length"="Median sample length 18", "x"=w499) -> ("median"=w498:dbl)  [unwired: 2 in, 1 out]
    n185 = Square(x=w498) -> (x^2=w506:dbl)
    n186 = Multiply(x=w498, y=0.1121) -> (x*y=w502:dbl)
    n187 = Multiply(x=w506, y=0.0243) -> (x*y=w503:dbl)
    n188 = Add(x=w502, y=w503) -> (x+y=w501:dbl)
    n189 = Add(x=-235.77, y=w501) -> (x+y=w465:dbl)
    n190 = case shown="True" "Autotune 9" {
      tunnel: w467 -> [w533 _]
      tunnel: [w522 w538] -> w472
      tunnel: w516 -> [_ w537]
      tunnel: "PID Gains 9" -> [w532 _]
      tunnel: "Reinitialize 9" -> [w529 _]
      tunnel: w517 -> [w531 w536]
      tunnel: w515 -> [_ w540]
      tunnel: w465 -> [w525 _]
      tunnel: "Set Point 3,4" -> [w524 _]
      frame False {
        # "This code is to have 'bumpless' transfer from autotuning"
        n191 = Not(x=w531) -> (.not. x?=w528:bool)
        n192 = And(x="Automatic 9", y=w528) -> (x .and. y?=w530:bool)
        n193 = call-poly <vilib>:"PID Advanced.vi"("setpoint"=w524, "auto? (T)"=w530, "manual control"="MV: 9", "process variable"=w525, "alpha"=10.0, "PID gains"=w532, "dt (s)"=w533, "reinitialize? (F)"=w529) -> ("output"=w522:dbl)  [unwired: 6 in, 1 out]
      }
      frame True {
        w543 = 10000 ("sample length")
        # "Buffering data for parameters estimation"
        n194 = call <vilib>:"Data Queue PtByPt.vi"("initial queue element"=w537, "initialize"=w536, "sample length"=w543, "input data point"=w537) -> ("Current Queue"=→"Control Output 9":dbl[])  [unwired: 3 in, 4 out]
        n195 = Select(t=0.0, s=w536, f="Excitation 9") -> (s? t:f=w541:dbl)
        n196 = Add(x=w540, y=w541) -> (x+y=w538:dbl)
        n197 = call <vilib>:"Data Queue PtByPt.vi"("initial queue element"=w538, "initialize"=w536, "sample length"=w543, "input data point"=w538) -> ("Current Queue"=→"Measurement 9":dbl[])  [unwired: 3 in, 4 out]
      }
    }
    n198 = feedback-in #6(w472, w513) -> ()
    n199 = Greater?(x=w465, y="M-3,4") -> (0:w455:bool)
    n200 = Add(x=w495, y=w483) -> (x+y=w484:dbl)
    n201 = Subtract(x=w495, y=w483) -> (x-y=w482:dbl)
    n202 = Equal?(x=w493, y=w472) -> (x = y?=w490:bool)
    n203 = Greater?(x=w472, y=w493) -> (0:w489:bool)
    n204 = Select(t=w494, s=w490, f=w489) -> (s? t:f=w470:bool)
    "PWM Output 9" <- w470
    n205 = call "Plant System.vi"("Integrator ?"=w512, "Plant Input"=w472, "dt (s)"=w467, "process parameters"=w510) -> ("Plant Output"=w511:dbl)  [unwired: 11 in]
    n206 = Increment(x="Set Point 3,4") -> (x+1=w488:dbl)
    n207 = Decrement(x="Set Point 3,4") -> (x-1=w487:dbl)
    n208 = Select(t=w484, s=w470, f=w482) -> (s? t:f=w497:dbl)
    n209 = Select(t=w488, s=w470, f=w487) -> (s? t:f=w486:dbl)
    n210 = Not(x=w470) -> (.not. x?=w469:bool)
    n211 = call-poly <vilib>:"DAQmx Create Virtual Channel.vi"("lines"=tag "cDAQ1Mod8/port0/line5", "line grouping"=w475) -> ("task out"=w477:refnum<k21>, "error out"=w476:errorcluster)  [unwired: 12 in]
    n212 = call-poly <vilib>:"DAQmx Create Virtual Channel.vi"("lines"=tag "cDAQ1Mod7/port0/line4", "line grouping"=w458) -> ("task out"=w460:refnum<k21>, "error out"=w459:errorcluster)  [unwired: 12 in]
    n213 = Build Array(w465, "Set Point 3,4", w486) -> (w485:dbl[])
    n214 = Initialize Array("INLET 3,4 ON/OFF 2", 1 ("dimension size")) -> (w434:bool[])
    n215 = Initialize Array(w469, 1 ("dimension size")) -> (w436:bool[])
    n216 = local write "MV: 9"(w472) -> ()
    n217 = Add(x=w492, y=w495) -> (x+y=w496:dbl)
    n218 = Build Array(w485) -> (→"Real time Data 3,4":dbl[][])
    n219 = call-poly <vilib>:"DAQmx Write.vi"("task/channels in"=w477, "auto start"=TRUE, "data"=w436, "error in"=w476) -> ("task out"=w479:refnum<k21>, "error out"=w480:errorcluster)  [unwired: 9 in, 1 out]
    n220 = call-poly <vilib>:"DAQmx Write.vi"("task/channels in"=w460, "auto start"=TRUE, "data"=w434, "error in"=w459) -> ("task out"=w462:refnum<k21>, "error out"=w463:errorcluster)  [unwired: 9 in, 1 out]
    n221 = call <vilib>:"DAQmx Clear Task.vi"("task in"=w479, "error in"=w480) -> ("error out"=w474:errorcluster)  [unwired: 13 in]
    n222 = call <vilib>:"DAQmx Clear Task.vi"("task in"=w462, "error in"=w463) -> ("error out"=w457:errorcluster)  [unwired: 13 in]
    n223 = call <vilib>:"Simple Error Handler.vi"("error in (no error)"=w474) -> ()  [unwired: 4 in, 5 out]
    n224 = call <vilib>:"Simple Error Handler.vi"("error in (no error)"=w457) -> ()  [unwired: 4 in, 5 out]
    n225 = call-poly <vilib>:"DAQmx Create Virtual Channel.vi"("lines"=tag "cDAQ1Mod8/port0/line7", "line grouping"=w446) -> ("task out"=w448:refnum<k21>, "error out"=w447:errorcluster)  [unwired: 12 in]
    n226 = call-poly <vilib>:"DAQmx Create Virtual Channel.vi"("lines"=tag "cDAQ1Mod7/port0/line6", "line grouping"=w438) -> ("task out"=w440:refnum<k21>, "error out"=w439:errorcluster)  [unwired: 12 in]
    n227 = call-poly <vilib>:"DAQmx Write.vi"("task/channels in"=w448, "auto start"=TRUE, "data"=w436, "error in"=w447) -> ("task out"=w450:refnum<k21>, "error out"=w451:errorcluster)  [unwired: 9 in, 1 out]
    n228 = call-poly <vilib>:"DAQmx Write.vi"("task/channels in"=w440, "auto start"=TRUE, "data"=w434, "error in"=w439) -> ("task out"=w442:refnum<k21>, "error out"=w443:errorcluster)  [unwired: 9 in, 1 out]
    n229 = call <vilib>:"DAQmx Clear Task.vi"("task in"=w450, "error in"=w451) -> ("error out"=w445:errorcluster)  [unwired: 13 in]
    n230 = call <vilib>:"DAQmx Clear Task.vi"("task in"=w442, "error in"=w443) -> ("error out"=w437:errorcluster)  [unwired: 13 in]
    n231 = call <vilib>:"Simple Error Handler.vi"("error in (no error)"=w445) -> ()  [unwired: 4 in, 5 out]
    n232 = call <vilib>:"Simple Error Handler.vi"("error in (no error)"=w437) -> ()  [unwired: 4 in, 5 out]
  }
  n233 = control-ref of="stop"() -> (w66:refnum<vi>)
  n234 = control-ref of="XYZAER"() -> (w57:refnum<vi>)
  n235 = Obtain Queue(element data type=0.0) -> (queue out=w5:refnum<queue>)  [unwired: 4 in, 2 out]
  n236 = while {
    shift-left: 0.0 ("Plant Output") -> [w610]
    shift-right: [w605] -> _
    tunnel: w34 -> [_]
    shift-right: [w591] -> _
    shift-left: 0.01 -> [w589]
    shift-right: [w563] -> _
    shift-left: TRUE -> [w588]
    shift-right: [w565] -> _
    shift-left: w31 -> [w587]
    shift-right: [w590] -> _
    shift-left: w31 -> [w586]
    tunnel: [w560] -> w30
    tunnel: [w546] -> w15
    tunnel: w5 -> [w544]
    stop <- "Stop 8" stop-if-true
    w551 = 1 items=["one channel for each line", "one channel for all lines"] ("line grouping")
    w560 = 0.05 ("Sampling Time dt (s)")
    w569 = 1 items=["one channel for each line", "one channel for all lines"] ("line grouping")
    w577 = 0.5 ("x")
    w604 = T7 {"static gain"=2.5, "lag (s)"=2.5, "deadtime (s)"=0.01, "load"=0.0, "deadband"=0.0, "sensor noise"=0.0, "initial PV"=30.0, "plant noise"=0.0}  # Process parameters
    w606 = FALSE  # Integrator ?
    # "C."
    # "Inlet 11"
    # "Exhaust 2"
    # "B."
    # "A."
    # "A.Output to PWM Logic \nB. Simulated Plant\nC. Draw Chart"
    # "Main PID Loop Control"
    n237 = Dequeue Element(queue=w544) -> (element=w545:dbl)  [unwired: 2 in, 3 out]
    n238 = Multiply(x=w560, y=1000.0) -> (x*y=w603:dbl)
    n239 = Not(x="Autotune 8") -> (.not. x?=w607:bool)
    n240 = feedback #7() -> (w612:bool)  [unwired: 1 in]
    n241 = feedback-in #7("Autotune 8") -> ()
    n242 = Wait Until Next ms Multiple(millisecond multiple=w603) -> ()  [unwired: 1 out]
    n243 = Exclusive Or(1:w612, 2:"Autotune 8") -> (0:w611:bool)
    n244 = feedback #8() -> (w609:dbl)  [unwired: 1 in]
    n245 = Multiply(x=w545, y=-1000.0) -> (x*y=w593:dbl)
    n246 = call <vilib>:"Median PtByPt.vi"("sample length"="Median sample length 17", "x"=w593) -> ("median"=w592:dbl)  [unwired: 2 in, 1 out]
    n247 = Square(x=w592) -> (x^2=w600:dbl)
    n248 = Multiply(x=w592, y=-7.5945) -> (x*y=w596:dbl)
    n249 = Multiply(x=w600, y=0.0612) -> (x*y=w597:dbl)
    n250 = Add(x=w596, y=w597) -> (x+y=w595:dbl)
    n251 = Add(x=143.72, y=w595) -> (x+y=w558:dbl)
    n252 = case shown="False" "Autotune 8" {
      tunnel: w560 -> [w627 _]
      tunnel: [w616 w632] -> w565
      tunnel: w610 -> [_ w631]
      tunnel: "PID Gains 8" -> [w626 _]
      tunnel: "Reinitialize 8" -> [w623 _]
      tunnel: w611 -> [w625 w630]
      tunnel: w609 -> [_ w634]
      tunnel: w558 -> [w619 _]
      tunnel: "Set Point 2" -> [w618 _]
      frame False {
        # "This code is to have 'bumpless' transfer from autotuning"
        n253 = Not(x=w625) -> (.not. x?=w622:bool)
        n254 = And(x="Automatic 8", y=w622) -> (x .and. y?=w624:bool)
        n255 = call-poly <vilib>:"PID Advanced.vi"("setpoint"=w618, "auto? (T)"=w624, "manual control"="MV: 8", "process variable"=w619, "alpha"=10.0, "PID gains"=w626, "dt (s)"=w627, "reinitialize? (F)"=w623) -> ("output"=w616:dbl)  [unwired: 6 in, 1 out]
      }
      frame True {
        w637 = 10000 ("sample length")
        # "Buffering data for parameters estimation"
        n256 = call <vilib>:"Data Queue PtByPt.vi"("initial queue element"=w631, "initialize"=w630, "sample length"=w637, "input data point"=w631) -> ("Current Queue"=→"Control Output 8":dbl[])  [unwired: 3 in, 4 out]
        n257 = Select(t=0.0, s=w630, f="Excitation 8") -> (s? t:f=w635:dbl)
        n258 = Add(x=w634, y=w635) -> (x+y=w632:dbl)
        n259 = call <vilib>:"Data Queue PtByPt.vi"("initial queue element"=w632, "initialize"=w630, "sample length"=w637, "input data point"=w632) -> ("Current Queue"=→"Measurement 8":dbl[])  [unwired: 3 in, 4 out]
      }
    }
    n260 = feedback-in #8(w565, w607) -> ()
    n261 = Greater?(x=w558, y="M-2") -> (0:w546:bool)
    n262 = Add(x=w589, y=w577) -> (x+y=w578:dbl)
    n263 = Subtract(x=w589, y=w577) -> (x-y=w576:dbl)
    n264 = Equal?(x=w587, y=w565) -> (x = y?=w584:bool)
    n265 = Greater?(x=w565, y=w587) -> (0:w583:bool)
    n266 = Select(t=w588, s=w584, f=w583) -> (s? t:f=w563:bool)
    "PWM Output 8" <- w563
    n267 = call "Plant System.vi"("Integrator ?"=w606, "Plant Input"=w565, "dt (s)"=w560, "process parameters"=w604) -> ("Plant Output"=w605:dbl)  [unwired: 11 in]
    n268 = Increment(x="Set Point 2") -> (x+1=w582:dbl)
    n269 = Decrement(x="Set Point 2") -> (x-1=w581:dbl)
    n270 = Select(t=w578, s=w563, f=w576) -> (s? t:f=w591:dbl)
    n271 = Select(t=w582, s=w563, f=w581) -> (s? t:f=w580:dbl)
    n272 = Not(x=w563) -> (.not. x?=w562:bool)
    n273 = call-poly <vilib>:"DAQmx Create Virtual Channel.vi"("lines"=tag "cDAQ1Mod1/port0/line6", "line grouping"=w569) -> ("task out"=w571:refnum<k21>, "error out"=w570:errorcluster)  [unwired: 12 in]
    n274 = call-poly <vilib>:"DAQmx Create Virtual Channel.vi"("lines"=tag "cDAQ1Mod2/port0/line6", "line grouping"=w551) -> ("task out"=w553:refnum<k21>, "error out"=w552:errorcluster)  [unwired: 12 in]
    n275 = Build Array(w558, "Set Point 2", w580) -> (w579:dbl[])
    n276 = Initialize Array("INLET 2 ON/OFF 2", 1 ("dimension size")) -> (w548:bool[])
    n277 = Initialize Array(w562, 1 ("dimension size")) -> (w566:bool[])
    n278 = local write "MV: 8"(w565) -> ()
    n279 = Add(x=w586, y=w589) -> (x+y=w590:dbl)
    n280 = Build Array(w579) -> (→"Real time Data 2":dbl[][])
    n281 = call-poly <vilib>:"DAQmx Write.vi"("task/channels in"=w571, "auto start"=TRUE, "data"=w566, "error in"=w570) -> ("task out"=w573:refnum<k21>, "error out"=w574:errorcluster)  [unwired: 9 in, 1 out]
    n282 = call-poly <vilib>:"DAQmx Write.vi"("task/channels in"=w553, "auto start"=TRUE, "data"=w548, "error in"=w552) -> ("task out"=w555:refnum<k21>, "error out"=w556:errorcluster)  [unwired: 9 in, 1 out]
    n283 = call <vilib>:"DAQmx Clear Task.vi"("task in"=w573, "error in"=w574) -> ("error out"=w568:errorcluster)  [unwired: 13 in]
    n284 = call <vilib>:"DAQmx Clear Task.vi"("task in"=w555, "error in"=w556) -> ("error out"=w550:errorcluster)  [unwired: 13 in]
    n285 = call <vilib>:"Simple Error Handler.vi"("error in (no error)"=w568) -> ()  [unwired: 4 in, 5 out]
    n286 = call <vilib>:"Simple Error Handler.vi"("error in (no error)"=w550) -> ()  [unwired: 4 in, 5 out]
  }
  n287 = Obtain Queue(element data type=0.0) -> (queue out=w4:refnum<queue>)  [unwired: 4 in, 2 out]
  n288 = while {
    shift-left: 0.0 ("Plant Output") -> [w704]
    shift-right: [w699] -> _
    shift-right: [w685] -> _
    shift-left: 0.01 -> [w683]
    shift-right: [w657] -> _
    shift-left: TRUE -> [w682]
    shift-right: [w659] -> _
    shift-left: w36 -> [w681]
    shift-right: [w684] -> _
    shift-left: w36 -> [w680]
    tunnel: [w640] -> w14
    tunnel: w4 -> [w638]
    stop <- "Stop 7" stop-if-true
    w645 = 1 items=["one channel for each line", "one channel for all lines"] ("line grouping")
    w654 = 0.05 ("Sampling Time dt (s)")
    w663 = 1 items=["one channel for each line", "one channel for all lines"] ("line grouping")
    w671 = 0.5 ("x")
    w698 = T7 {"static gain"=2.5, "lag (s)"=2.5, "deadtime (s)"=0.01, "load"=0.0, "deadband"=0.0, "sensor noise"=0.0, "initial PV"=30.0, "plant noise"=0.0}  # Process parameters
    w700 = FALSE  # Integrator ?
    # "C."
    # "Inlet 11"
    # "Exhaust 7"
    # "B."
    # "A."
    # "A.Output to PWM Logic \nB. Simulated Plant\nC. Draw Chart"
    # "Main PID Loop Control"
    n289 = Dequeue Element(queue=w638) -> (element=w639:dbl)  [unwired: 2 in, 3 out]
    n290 = Multiply(x=w654, y=1000.0) -> (x*y=w697:dbl)
    n291 = Not(x="Autotune 7") -> (.not. x?=w701:bool)
    n292 = feedback #9() -> (w706:bool)  [unwired: 1 in]
    n293 = feedback-in #9("Autotune 7") -> ()
    n294 = Wait Until Next ms Multiple(millisecond multiple=w697) -> ()  [unwired: 1 out]
    n295 = Exclusive Or(1:w706, 2:"Autotune 7") -> (0:w705:bool)
    n296 = feedback #10() -> (w703:dbl)  [unwired: 1 in]
    n297 = Multiply(x=w639, y=-1000.0) -> (x*y=w687:dbl)
    n298 = call <vilib>:"Median PtByPt.vi"("sample length"="Median sample length 16", "x"=w687) -> ("median"=w686:dbl)  [unwired: 2 in, 1 out]
    n299 = Square(x=w686) -> (x^2=w694:dbl)
    n300 = Multiply(x=w686, y=-0.6707) -> (x*y=w690:dbl)
    n301 = Multiply(x=w694, y=0.0015) -> (x*y=w691:dbl)
    n302 = Add(x=w690, y=w691) -> (x+y=w689:dbl)
    n303 = Add(x=-0.8771, y=w689) -> (x+y=w652:dbl)
    n304 = case shown="False" "Autotune 7" {
      tunnel: w654 -> [w721 _]
      tunnel: [w710 w726] -> w659
      tunnel: w704 -> [_ w725]
      tunnel: "PID Gains 7" -> [w720 _]
      tunnel: "Reinitialize 7" -> [w717 _]
      tunnel: w705 -> [w719 w724]
      tunnel: w703 -> [_ w728]
      tunnel: w652 -> [w713 _]
      tunnel: "Set Point 7" -> [w712 _]
      frame False {
        # "This code is to have 'bumpless' transfer from autotuning"
        n305 = Not(x=w719) -> (.not. x?=w716:bool)
        n306 = And(x="Automatic 7", y=w716) -> (x .and. y?=w718:bool)
        n307 = call-poly <vilib>:"PID Advanced.vi"("setpoint"=w712, "auto? (T)"=w718, "manual control"="MV: 7", "process variable"=w713, "alpha"=10.0, "PID gains"=w720, "dt (s)"=w721, "reinitialize? (F)"=w717) -> ("output"=w710:dbl)  [unwired: 6 in, 1 out]
      }
      frame True {
        w731 = 10000 ("sample length")
        # "Buffering data for parameters estimation"
        n308 = call <vilib>:"Data Queue PtByPt.vi"("initial queue element"=w725, "initialize"=w724, "sample length"=w731, "input data point"=w725) -> ("Current Queue"=→"Control Output 7":dbl[])  [unwired: 3 in, 4 out]
        n309 = Select(t=0.0, s=w724, f="Excitation 7") -> (s? t:f=w729:dbl)
        n310 = Add(x=w728, y=w729) -> (x+y=w726:dbl)
        n311 = call <vilib>:"Data Queue PtByPt.vi"("initial queue element"=w726, "initialize"=w724, "sample length"=w731, "input data point"=w726) -> ("Current Queue"=→"Measurement 7":dbl[])  [unwired: 3 in, 4 out]
      }
    }
    n312 = feedback-in #10(w659, w701) -> ()
    n313 = Greater?(x=w652, y="M-7") -> (0:w640:bool)
    n314 = Add(x=w683, y=w671) -> (x+y=w672:dbl)
    n315 = Subtract(x=w683, y=w671) -> (x-y=w670:dbl)
    n316 = Equal?(x=w681, y=w659) -> (x = y?=w678:bool)
    n317 = Greater?(x=w659, y=w681) -> (0:w677:bool)
    n318 = Select(t=w682, s=w678, f=w677) -> (s? t:f=w657:bool)
    "PWM Output 7" <- w657
    n319 = call "Plant System.vi"("Integrator ?"=w700, "Plant Input"=w659, "dt (s)"=w654, "process parameters"=w698) -> ("Plant Output"=w699:dbl)  [unwired: 11 in]
    n320 = Increment(x="Set Point 7") -> (x+1=w676:dbl)
    n321 = Decrement(x="Set Point 7") -> (x-1=w675:dbl)
    n322 = Select(t=w672, s=w657, f=w670) -> (s? t:f=w685:dbl)
    n323 = Select(t=w676, s=w657, f=w675) -> (s? t:f=w674:dbl)
    n324 = Not(x=w657) -> (.not. x?=w656:bool)
    n325 = call-poly <vilib>:"DAQmx Create Virtual Channel.vi"("lines"=tag "cDAQ1Mod8/port0/line4", "line grouping"=w663) -> ("task out"=w665:refnum<k21>, "error out"=w664:errorcluster)  [unwired: 12 in]
    n326 = call-poly <vilib>:"DAQmx Create Virtual Channel.vi"("lines"=tag "cDAQ1Mod7/port0/line3", "line grouping"=w645) -> ("task out"=w647:refnum<k21>, "error out"=w646:errorcluster)  [unwired: 12 in]
    n327 = Build Array(w652, "Set Point 7", w674) -> (w673:dbl[])
    n328 = Initialize Array("INLET 7 ON/OFF 2", 1 ("dimension size")) -> (w642:bool[])
    n329 = Initialize Array(w656, 1 ("dimension size")) -> (w660:bool[])
    n330 = local write "MV: 7"(w659) -> ()
    n331 = Add(x=w680, y=w683) -> (x+y=w684:dbl)
    n332 = Build Array(w673) -> (→"Real time Data 7":dbl[][])
    n333 = call-poly <vilib>:"DAQmx Write.vi"("task/channels in"=w665, "auto start"=TRUE, "data"=w660, "error in"=w664) -> ("task out"=w667:refnum<k21>, "error out"=w668:errorcluster)  [unwired: 9 in, 1 out]
    n334 = call-poly <vilib>:"DAQmx Write.vi"("task/channels in"=w647, "auto start"=TRUE, "data"=w642, "error in"=w646) -> ("task out"=w649:refnum<k21>, "error out"=w650:errorcluster)  [unwired: 9 in, 1 out]
    n335 = call <vilib>:"DAQmx Clear Task.vi"("task in"=w667, "error in"=w668) -> ("error out"=w662:errorcluster)  [unwired: 13 in]
    n336 = call <vilib>:"DAQmx Clear Task.vi"("task in"=w649, "error in"=w650) -> ("error out"=w644:errorcluster)  [unwired: 13 in]
    n337 = call <vilib>:"Simple Error Handler.vi"("error in (no error)"=w662) -> ()  [unwired: 4 in, 5 out]
    n338 = call <vilib>:"Simple Error Handler.vi"("error in (no error)"=w644) -> ()  [unwired: 4 in, 5 out]
  }
  n339 = Obtain Queue(element data type=0.0) -> (queue out=w10:refnum<queue>)  [unwired: 4 in, 2 out]
  n340 = while {
    shift-left: 0.0 ("Plant Output") -> [w832]
    shift-right: [w827] -> _
    shift-right: [w813] -> _
    shift-left: 0.01 -> [w811]
    shift-right: [w786] -> _
    shift-left: TRUE -> [w810]
    shift-right: [w788] -> _
    shift-left: w83 -> [w809]
    shift-right: [w812] -> _
    shift-left: w83 -> [w808]
    tunnel: [w780] -> w1
    tunnel: w12 -> [w758]
    tunnel: w10 -> [w757]
    tunnel: w8 -> [w756]
    tunnel: w5 -> [w753]
    tunnel: w4 -> [w752]
    stop <- "Stop" stop-if-true
    w737 = 1 items=["one channel for each line", "one channel for all lines"] ("line grouping")
    w745 = 1 items=["one channel for each line", "one channel for all lines"] ("line grouping")
    w773 = 1 items=["one channel for each line", "one channel for all lines"] ("line grouping")
    w783 = 0.05 ("Sampling Time dt (s)")
    w791 = 1 items=["one channel for each line", "one channel for all lines"] ("line grouping")
    w799 = 0.5 ("x")
    w826 = T7 {"static gain"=2.5, "lag (s)"=2.5, "deadtime (s)"=0.01, "load"=0.0, "deadband"=0.0, "sensor noise"=0.0, "initial PV"=30.0, "plant noise"=0.0}  # Process parameters
    w828 = FALSE  # Integrator ?
    # "Inlet 11"
    # "Exhaust 12"
    # "C."
    # "Inlet 11"
    # "Exhaust 11"
    # "B."
    # "A."
    # "A.Output to PWM Logic \nB. Simulated Plant\nC. Draw Chart"
    # "Main PID Loop Control"
    n341 = call-poly <vilib>:"DAQmx Read.vi"("task/channels in"=refnum<k21> "1_4_2_7_6_5") -> ("data"=w763:dbl[])  [unwired: 12 in, 2 out]
    n342 = Index Array(array=w763, index=0) -> (element=w759:dbl)
    n343 = Index Array(array=w763, index=1) -> (element=w760:dbl)
    n344 = Index Array(array=w763, index=2) -> (element=w755:dbl)
    n345 = Index Array(array=w763, index=5) -> (element=w733:dbl)
    n346 = Index Array(array=w763, index=4) -> (element=w761:dbl)
    n347 = Index Array(array=w763, index=3) -> (element=w754:dbl)
    n348 = Enqueue Element(queue=w757, element=w759) -> ()  [unwired: 2 in, 3 out]
    n349 = Enqueue Element(queue=w753, element=w755) -> ()  [unwired: 2 in, 3 out]
    n350 = Multiply(x=w783, y=1000.0) -> (x*y=w825:dbl)
    n351 = Enqueue Element(queue=w756, element=w760) -> ()  [unwired: 2 in, 3 out]
    n352 = call <vilib>:"Butterworth Filter PtByPt.vi"("x"=w733) -> ("Filtered x"=w732:dbl)  [unwired: 8 in, 1 out]
    n353 = Not(x="Autotune") -> (.not. x?=w829:bool)
    n354 = feedback #11() -> (w834:bool)  [unwired: 1 in]
    n355 = feedback-in #11("Autotune") -> ()
    n356 = Enqueue Element(queue=w752, element=w754) -> ()  [unwired: 2 in, 3 out]
    n357 = Wait Until Next ms Multiple(millisecond multiple=w825) -> ()  [unwired: 1 out]
    n358 = Exclusive Or(1:w834, 2:"Autotune") -> (0:w833:bool)
    n359 = feedback #12() -> (w831:dbl)  [unwired: 1 in]
    n360 = Enqueue Element(queue=w758, element=w761) -> ()  [unwired: 2 in, 3 out]
    n361 = Multiply(x=w732, y=-1000.0) -> (x*y=w815:dbl)
    n362 = call <vilib>:"Median PtByPt.vi"("sample length"="Median sample length", "x"=w815) -> ("median"=w814:dbl)  [unwired: 2 in, 1 out]
    n363 = Square(x=w814) -> (x^2=w822:dbl)
    n364 = Multiply(x=w814, y=-39.646) -> (x*y=w818:dbl)
    n365 = Multiply(x=w822, y=0.2324) -> (x*y=w819:dbl)
    n366 = Add(x=w818, y=w819) -> (x+y=w817:dbl)
    n367 = Add(x=1678.0, y=w817) -> (x+y=w781:dbl)
    n368 = case shown="False" "Autotune" {
      tunnel: w783 -> [w849 _]
      tunnel: [w838 w854] -> w788
      tunnel: w832 -> [_ w853]
      tunnel: "PID Gains" -> [w848 _]
      tunnel: "Reinitialize" -> [w845 _]
      tunnel: w833 -> [w847 w852]
      tunnel: w831 -> [_ w856]
      tunnel: w781 -> [w841 _]
      tunnel: "Set Point 11,12" -> [w840 _]
      frame False {
        # "This code is to have 'bumpless' transfer from autotuning"
        n369 = Not(x=w847) -> (.not. x?=w844:bool)
        n370 = And(x="Automatic", y=w844) -> (x .and. y?=w846:bool)
        n371 = call-poly <vilib>:"PID Advanced.vi"("setpoint"=w840, "auto? (T)"=w846, "manual control"="MV:", "process variable"=w841, "alpha"=10.0, "PID gains"=w848, "dt (s)"=w849, "reinitialize? (F)"=w845) -> ("output"=w838:dbl)  [unwired: 6 in, 1 out]
      }
      frame True {
        w859 = 10000 ("sample length")
        # "Buffering data for parameters estimation"
        n372 = call <vilib>:"Data Queue PtByPt.vi"("initial queue element"=w853, "initialize"=w852, "sample length"=w859, "input data point"=w853) -> ("Current Queue"=→"Control Output":dbl[])  [unwired: 3 in, 4 out]
        n373 = Select(t=0.0, s=w852, f="Excitation") -> (s? t:f=w857:dbl)
        n374 = Add(x=w856, y=w857) -> (x+y=w854:dbl)
        n375 = call <vilib>:"Data Queue PtByPt.vi"("initial queue element"=w854, "initialize"=w852, "sample length"=w859, "input data point"=w854) -> ("Current Queue"=→"Measurement":dbl[])  [unwired: 3 in, 4 out]
      }
    }
    n376 = feedback-in #12(w788, w829) -> ()
    n377 = Greater?(x=w781, y="M-11,12") -> (0:w780:bool)
    n378 = Add(x=w811, y=w799) -> (x+y=w800:dbl)
    n379 = Subtract(x=w811, y=w799) -> (x-y=w798:dbl)
    n380 = Equal?(x=w809, y=w788) -> (x = y?=w806:bool)
    n381 = Greater?(x=w788, y=w809) -> (0:w805:bool)
    n382 = Select(t=w810, s=w806, f=w805) -> (s? t:f=w786:bool)
    "PWM Output" <- w786
    n383 = call "Plant System.vi"("Integrator ?"=w828, "Plant Input"=w788, "dt (s)"=w783, "process parameters"=w826) -> ("Plant Output"=w827:dbl)  [unwired: 11 in]
    n384 = Increment(x="Set Point 11,12") -> (x+1=w804:dbl)
    n385 = Decrement(x="Set Point 11,12") -> (x-1=w803:dbl)
    n386 = Select(t=w800, s=w786, f=w798) -> (s? t:f=w813:dbl)
    n387 = Select(t=w804, s=w786, f=w803) -> (s? t:f=w802:dbl)
    n388 = Not(x=w786) -> (.not. x?=w785:bool)
    n389 = call-poly <vilib>:"DAQmx Create Virtual Channel.vi"("lines"=tag "cDAQ1Mod1/port0/line2", "line grouping"=w791) -> ("task out"=w793:refnum<k21>, "error out"=w792:errorcluster)  [unwired: 12 in]
    n390 = call-poly <vilib>:"DAQmx Create Virtual Channel.vi"("lines"=tag "cDAQ1Mod2/port0/line2", "line grouping"=w773) -> ("task out"=w775:refnum<k21>, "error out"=w774:errorcluster)  [unwired: 12 in]
    n391 = Build Array(w781, "Set Point 11,12", w802) -> (w801:dbl[])
    n392 = Initialize Array("INLET", 1 ("dimension size")) -> (w734:bool[])
    n393 = Initialize Array(w785, 1 ("dimension size")) -> (w735:bool[])
    n394 = call-poly <vilib>:"DAQmx Create Virtual Channel.vi"("lines"=tag "cDAQ1Mod8/port0/line2", "line grouping"=w745) -> ("task out"=w747:refnum<k21>, "error out"=w746:errorcluster)  [unwired: 12 in]
    n395 = call-poly <vilib>:"DAQmx Create Virtual Channel.vi"("lines"=tag "cDAQ1Mod7/port0/line1", "line grouping"=w737) -> ("task out"=w739:refnum<k21>, "error out"=w738:errorcluster)  [unwired: 12 in]
    n396 = local write "MV:"(w788) -> ()
    n397 = Add(x=w808, y=w811) -> (x+y=w812:dbl)
    n398 = Build Array(w801) -> (→"Real time Data -11,12":dbl[][])
    n399 = call-poly <vilib>:"DAQmx Write.vi"("task/channels in"=w793, "auto start"=TRUE, "data"=w735, "error in"=w792) -> ("task out"=w795:refnum<k21>, "error out"=w796:errorcluster)  [unwired: 9 in, 1 out]
    n400 = call-poly <vilib>:"DAQmx Write.vi"("task/channels in"=w775, "auto start"=TRUE, "data"=w734, "error in"=w774) -> ("task out"=w777:refnum<k21>, "error out"=w778:errorcluster)  [unwired: 9 in, 1 out]
    n401 = call-poly <vilib>:"DAQmx Write.vi"("task/channels in"=w747, "auto start"=TRUE, "data"=w735, "error in"=w746) -> ("task out"=w749:refnum<k21>, "error out"=w750:errorcluster)  [unwired: 9 in, 1 out]
    n402 = call-poly <vilib>:"DAQmx Write.vi"("task/channels in"=w739, "auto start"=TRUE, "data"=w734, "error in"=w738) -> ("task out"=w741:refnum<k21>, "error out"=w742:errorcluster)  [unwired: 9 in, 1 out]
    n403 = call <vilib>:"DAQmx Clear Task.vi"("task in"=w795, "error in"=w796) -> ("error out"=w790:errorcluster)  [unwired: 13 in]
    n404 = call <vilib>:"DAQmx Clear Task.vi"("task in"=w777, "error in"=w778) -> ("error out"=w772:errorcluster)  [unwired: 13 in]
    n405 = call <vilib>:"DAQmx Clear Task.vi"("task in"=w749, "error in"=w750) -> ("error out"=w744:errorcluster)  [unwired: 13 in]
    n406 = call <vilib>:"DAQmx Clear Task.vi"("task in"=w741, "error in"=w742) -> ("error out"=w736:errorcluster)  [unwired: 13 in]
    n407 = call <vilib>:"Simple Error Handler.vi"("error in (no error)"=w790) -> ()  [unwired: 4 in, 5 out]
    n408 = call <vilib>:"Simple Error Handler.vi"("error in (no error)"=w772) -> ()  [unwired: 4 in, 5 out]
    n409 = call <vilib>:"Simple Error Handler.vi"("error in (no error)"=w744) -> ()  [unwired: 4 in, 5 out]
    n410 = call <vilib>:"Simple Error Handler.vi"("error in (no error)"=w736) -> ()  [unwired: 4 in, 5 out]
  }
  n411 = while {
    shift-left: 0.0 ("Plant Output") -> [w944]
    shift-right: [w939] -> _
    tunnel: w22 -> [_]
    shift-right: [w925] -> _
    shift-left: 0.01 -> [w923]
    shift-right: [w898] -> _
    shift-left: TRUE -> [w922]
    shift-right: [w900] -> _
    shift-left: w19 -> [w921]
    shift-right: [w924] -> _
    shift-left: w19 -> [w920]
    tunnel: [w895] -> w18
    tunnel: [w882] -> w3
    tunnel: w10 -> [w880]
    stop <- "Stop 12" stop-if-true
    w865 = 1 items=["one channel for each line", "one channel for all lines"] ("line grouping")
    w873 = 1 items=["one channel for each line", "one channel for all lines"] ("line grouping")
    w886 = 1 items=["one channel for each line", "one channel for all lines"] ("line grouping")
    w895 = 0.05 ("Sampling Time dt (s)")
    w903 = 1 items=["one channel for each line", "one channel for all lines"] ("line grouping")
    w911 = 0.5 ("x")
    w938 = T7 {"static gain"=2.5, "lag (s)"=2.5, "deadtime (s)"=0.01, "load"=0.0, "deadband"=0.0, "sensor noise"=0.0, "initial PV"=30.0, "plant noise"=0.0}  # Process parameters
    w940 = FALSE  # Integrator ?
    # "Inlet 11"
    # "Exhaust 5"
    # "C."
    # "Inlet 11"
    # "Exhaust 1"
    # "B."
    # "A."
    # "A.Output to PWM Logic \nB. Simulated Plant\nC. Draw Chart"
    # "Main PID Loop Control"
    n412 = Dequeue Element(queue=w880) -> (element=w881:dbl)  [unwired: 2 in, 3 out]
    n413 = Multiply(x=w895, y=1000.0) -> (x*y=w937:dbl)
    n414 = Not(x="Autotune 12") -> (.not. x?=w941:bool)
    n415 = feedback #13() -> (w946:bool)  [unwired: 1 in]
    n416 = feedback-in #13("Autotune 12") -> ()
    n417 = Wait Until Next ms Multiple(millisecond multiple=w937) -> ()  [unwired: 1 out]
    n418 = Exclusive Or(1:w946, 2:"Autotune 12") -> (0:w945:bool)
    n419 = feedback #14() -> (w943:dbl)  [unwired: 1 in]
    n420 = Multiply(x=w881, y=-1000.0) -> (x*y=w927:dbl)
    n421 = call <vilib>:"Median PtByPt.vi"("sample length"="Median sample length 21", "x"=w927) -> ("median"=w926:dbl)  [unwired: 2 in, 1 out]
    n422 = Square(x=w926) -> (x^2=w934:dbl)
    n423 = Multiply(x=w926, y=2.7367) -> (x*y=w930:dbl)
    n424 = Multiply(x=w934, y=0.0108) -> (x*y=w931:dbl)
    n425 = Add(x=w930, y=w931) -> (x+y=w929:dbl)
    n426 = Add(x=-331.61, y=w929) -> (x+y=w893:dbl)
    n427 = case shown="True" "Autotune 12" {
      tunnel: w895 -> [w961 _]
      tunnel: [w950 w966] -> w900
      tunnel: w944 -> [_ w965]
      tunnel: "PID Gains 12" -> [w960 _]
      tunnel: "Reinitialize 12" -> [w957 _]
      tunnel: w945 -> [w959 w964]
      tunnel: w943 -> [_ w968]
      tunnel: w893 -> [w953 _]
      tunnel: "Set Point 1,5" -> [w952 _]
      frame False {
        # "This code is to have 'bumpless' transfer from autotuning"
        n428 = Not(x=w959) -> (.not. x?=w956:bool)
        n429 = And(x="Automatic 12", y=w956) -> (x .and. y?=w958:bool)
        n430 = call-poly <vilib>:"PID Advanced.vi"("setpoint"=w952, "auto? (T)"=w958, "manual control"="MV: 12", "process variable"=w953, "alpha"=10.0, "PID gains"=w960, "dt (s)"=w961, "reinitialize? (F)"=w957) -> ("output"=w950:dbl)  [unwired: 6 in, 1 out]
      }
      frame True {
        w971 = 10000 ("sample length")
        # "Buffering data for parameters estimation"
        n431 = call <vilib>:"Data Queue PtByPt.vi"("initial queue element"=w965, "initialize"=w964, "sample length"=w971, "input data point"=w965) -> ("Current Queue"=→"Control Output 12":dbl[])  [unwired: 3 in, 4 out]
        n432 = Select(t=0.0, s=w964, f="Excitation 12") -> (s? t:f=w969:dbl)
        n433 = Add(x=w968, y=w969) -> (x+y=w966:dbl)
        n434 = call <vilib>:"Data Queue PtByPt.vi"("initial queue element"=w966, "initialize"=w964, "sample length"=w971, "input data point"=w966) -> ("Current Queue"=→"Measurement 12":dbl[])  [unwired: 3 in, 4 out]
      }
    }
    n435 = feedback-in #14(w900, w941) -> ()
    n436 = Greater?(x=w893, y="M-1,5") -> (0:w882:bool)
    n437 = Add(x=w923, y=w911) -> (x+y=w912:dbl)
    n438 = Subtract(x=w923, y=w911) -> (x-y=w910:dbl)
    n439 = Equal?(x=w921, y=w900) -> (x = y?=w918:bool)
    n440 = Greater?(x=w900, y=w921) -> (0:w917:bool)
    n441 = Select(t=w922, s=w918, f=w917) -> (s? t:f=w898:bool)
    "PWM Output 12" <- w898
    n442 = call "Plant System.vi"("Integrator ?"=w940, "Plant Input"=w900, "dt (s)"=w895, "process parameters"=w938) -> ("Plant Output"=w939:dbl)  [unwired: 11 in]
    n443 = Increment(x="Set Point 1,5") -> (x+1=w916:dbl)
    n444 = Decrement(x="Set Point 1,5") -> (x-1=w915:dbl)
    n445 = Select(t=w912, s=w898, f=w910) -> (s? t:f=w925:dbl)
    n446 = Select(t=w916, s=w898, f=w915) -> (s? t:f=w914:dbl)
    n447 = Not(x=w898) -> (.not. x?=w897:bool)
    n448 = call-poly <vilib>:"DAQmx Create Virtual Channel.vi"("lines"=tag "cDAQ1Mod1/port0/line7", "line grouping"=w903) -> ("task out"=w905:refnum<k21>, "error out"=w904:errorcluster)  [unwired: 12 in]
    n449 = call-poly <vilib>:"DAQmx Create Virtual Channel.vi"("lines"=tag "cDAQ1Mod2/port0/line7", "line grouping"=w886) -> ("task out"=w888:refnum<k21>, "error out"=w887:errorcluster)  [unwired: 12 in]
    n450 = Build Array(w893, "Set Point 1,5", w914) -> (w913:dbl[])
    n451 = Initialize Array("INLET 1,5 ON/OFF 3", 1 ("dimension size")) -> (w883:bool[])
    n452 = Initialize Array(w897, 1 ("dimension size")) -> (w860:bool[])
    n453 = local write "MV: 12"(w900) -> ()
    n454 = Add(x=w920, y=w923) -> (x+y=w924:dbl)
    n455 = Build Array(w913) -> (→"Real time Data 1,5":dbl[][])
    n456 = call-poly <vilib>:"DAQmx Write.vi"("task/channels in"=w905, "auto start"=TRUE, "data"=w860, "error in"=w904) -> ("task out"=w907:refnum<k21>, "error out"=w908:errorcluster)  [unwired: 9 in, 1 out]
    n457 = call-poly <vilib>:"DAQmx Write.vi"("task/channels in"=w888, "auto start"=TRUE, "data"=w883, "error in"=w887) -> ("task out"=w890:refnum<k21>, "error out"=w891:errorcluster)  [unwired: 9 in, 1 out]
    n458 = call <vilib>:"DAQmx Clear Task.vi"("task in"=w907, "error in"=w908) -> ("error out"=w902:errorcluster)  [unwired: 13 in]
    n459 = call <vilib>:"DAQmx Clear Task.vi"("task in"=w890, "error in"=w891) -> ("error out"=w885:errorcluster)  [unwired: 13 in]
    n460 = call <vilib>:"Simple Error Handler.vi"("error in (no error)"=w902) -> ()  [unwired: 4 in, 5 out]
    n461 = call <vilib>:"Simple Error Handler.vi"("error in (no error)"=w885) -> ()  [unwired: 4 in, 5 out]
    n462 = call-poly <vilib>:"DAQmx Create Virtual Channel.vi"("lines"=tag "cDAQ1Mod1/port0/line5", "line grouping"=w873) -> ("task out"=w875:refnum<k21>, "error out"=w874:errorcluster)  [unwired: 12 in]
    n463 = call-poly <vilib>:"DAQmx Create Virtual Channel.vi"("lines"=tag "cDAQ1Mod2/port0/line5", "line grouping"=w865) -> ("task out"=w867:refnum<k21>, "error out"=w866:errorcluster)  [unwired: 12 in]
    n464 = Initialize Array("INLET 1,5 ON/OFF 3", 1 ("dimension size")) -> (w862:bool[])
    n465 = call-poly <vilib>:"DAQmx Write.vi"("task/channels in"=w875, "auto start"=TRUE, "data"=w860, "error in"=w874) -> ("task out"=w877:refnum<k21>, "error out"=w878:errorcluster)  [unwired: 9 in, 1 out]
    n466 = call-poly <vilib>:"DAQmx Write.vi"("task/channels in"=w867, "auto start"=TRUE, "data"=w862, "error in"=w866) -> ("task out"=w869:refnum<k21>, "error out"=w870:errorcluster)  [unwired: 9 in, 1 out]
    n467 = call <vilib>:"DAQmx Clear Task.vi"("task in"=w877, "error in"=w878) -> ("error out"=w872:errorcluster)  [unwired: 13 in]
    n468 = call <vilib>:"DAQmx Clear Task.vi"("task in"=w869, "error in"=w870) -> ("error out"=w864:errorcluster)  [unwired: 13 in]
    n469 = call <vilib>:"Simple Error Handler.vi"("error in (no error)"=w872) -> ()  [unwired: 4 in, 5 out]
    n470 = call <vilib>:"Simple Error Handler.vi"("error in (no error)"=w864) -> ()  [unwired: 4 in, 5 out]
  }
  n471 = Compound Arithmetic op=OR(w1, w2, w3, w16, w15, w14) -> (w17:bool)
  "?" <- w17
  n472 = case shown="True" w17 {
    frame False {
    }
    frame True {
      n473 = call <vilib>:"Beep.vi"("use system alert? (T)"=FALSE, "duration (msec)"=u32 2000, "frequency (Hz)"=u32 15000) -> ()  [unwired: 9 in]
    }
  }
  n474 = control-ref of="PnoData"() -> (w48:refnum<vi>)
  n475 = call <instrlib>:"PDI data xyzaer loop.vi"("Data Ready Refnum"=w48, "FrameCount Ctl Ref"=w58, "error in (no error)"=w68, "xyzaer array\nRefnum"=w57, "Stop Ctl Ref"=w66, "pDev"=w67) -> ("error out"=w55:errorcluster, "Loop Iter"=w59:i32, "dup pDev"=w56:u32)  [unwired: 3 out]
  n476 = local write "Loop Iter"(w59) -> ()
  n477 = local write "Stop 9"(w28) -> ()
  n478 = local write "Stop 12"(w22) -> ()
  n479 = call <instrlib>:"PDI action stopcont.vi"("error in (no error)"=w55, "pDev"=w56) -> ("error out"=w64:errorcluster, "Running"=w69:bool, "dup pDev"=w70:u32)  [unwired: 7 out]
  n480 = local write "Stop 8"(w34) -> ()
  n481 = local write "Stop 7"(FALSE ("Stop")) -> ()
  n482 = local write "Running"(w69) -> ()
  n483 = case shown="No Error" w55 {
    tunnel: w63 -> [w975 _]
    frame No Error {
      # "Success up to here"
      n484 = call "Elapsed Time"("Set Start Time (s)"=w975) -> ("Present Text"=w977:string, "Elapsed Time Text"=w976:string)  [unwired: 4 in, 13 out]
      n485 = local write "Stop Time Text"(w977) -> ()
      n486 = local write "Elapsed Time Text"(w976) -> ()
    }
    frame Error {
      # "Error somewhere;\nStop Time is irrelevant"
    }
  }
  n487 = while {
    tunnel: w28 -> [_]
    tunnel: w24 -> [_]
    stop <- w993 stop-if-true
    w978 = 0.05 ("Sampling Time dt (s)")
    # "If dT and deadtime have similar values, the identification could evaluate deadtime as zero and this generates proportional gain equal to Inf. This code avoid gain changes in this situations."
    # "Autotuning Loop"
    n488 = local read "Control Output 9"() -> (w995:dbl[])
    n489 = local read "Measurement 9"() -> (w994:dbl[])
    n490 = Multiply(x=w978, y=1000.0) -> (x*y=w980:dbl)
    n491 = Wait Until Next ms Multiple(millisecond multiple=w980) -> ()  [unwired: 1 out]
    n492 = case shown="\"Internal Model Control\"" "Control 9" {
      tunnel: w995 -> [w1004 w1012 w1021 w1030]
      tunnel: w994 -> [w1003 w1011 w1020 w1029]
      tunnel: [w1002 w1010 w1019 w1028] -> w982
      tunnel: [w1001 w1009 w1018 w1027] -> w981
      tunnel: w978 -> [w1000 w1008 w1017 w1026]
      tunnel: [w999 w1007 w1016 w1025] -> w983
      tunnel: [w998 w1006 w1015 w1024] -> w985
      tunnel: "Type of controller 9" -> [w997 w1005 w1014 w1023]
      frame "Ziegler-Nichols", Default {
        n493 = call-poly <vilib>:"PID Autotuning Design.vi"("Ziegler-Nichols Speed"="Ziegler-Nichols speed 9", "Type of Controller"=w997, "dt (s)"=w1000, "Response signal"=w1003, "Stimulus signal"=w1004) -> ("PID gains"=w998:T3, "response operating point"=w1001:dbl, "stimulus operating point"=w1002:dbl, "Plant Parameters"=w999:T5)  [unwired: 3 in]
      }
      frame "Cohen-Coon" {
        n494 = call-poly <vilib>:"PID Autotuning Design.vi"("Type of Controller"=w1005, "dt (s)"=w1008, "Response signal"=w1011, "Stimulus signal"=w1012) -> ("PID gains"=w1006:T3, "response offset"=w1009:dbl, "stimulus offset"=w1010:dbl, "Plant Parameters"=w1007:T5)  [unwired: 4 in]
      }
      frame "Chien-Hrones-Reswick" {
        n495 = call-poly <vilib>:"PID Autotuning Design.vi"("Tuning specifications"="Tuning specifications 9", "Type of Controller"=w1014, "dt (s)"=w1017, "Response signal"=w1020, "Stimulus signal"=w1021) -> ("PID gains"=w1015:T3, "response offset"=w1018:dbl, "stimulus offset"=w1019:dbl, "Plant Parameters"=w1016:T5)  [unwired: 3 in]
      }
      frame "Internal Model Control" {
        n496 = call-poly <vilib>:"PID Autotuning Design.vi"("Desired Time Constant (tau_c)"="Multiplicative factor 9", "Type of Controller"=w1023, "dt (s)"=w1026, "Response signal"=w1029, "Stimulus signal"=w1030) -> ("PID gains"=w1024:T3, "response offset"=w1027:dbl, "stimulus offset"=w1028:dbl, "Plant Parameters"=w1025:T5)  [unwired: 3 in]
      }
    }
    "Identified Plant Parameters 9" <- w983
    "Response operating point 9" <- w981
    "Stimulus operating point 9" <- w982
    n497 = Unbundle(w985) -> ("proportional gain (Kc)"=w988:dbl)  [unwired: 2 out]
    n498 = Equal?(x=w988, y=inf) -> (x = y?=w987:bool)
    n499 = feedback #15() -> (w986:T3)  [unwired: 1 in]
    n500 = Select(t=w986, s=w987, f=w985) -> (s? t:f=w984:T3)
    "Tuned PID gains 9" <- w984
    n501 = feedback-in #15(w984) -> ()
    n502 = case shown="True" "Accept gain 9" {
      tunnel: w984 -> [_ w1031]
      frame False {
      }
      frame True {
        n503 = local write "PID Gains 9"(w1031) -> ()
      }
    }
    n504 = local read "Stop 9"() -> (w993:bool)
  }
  n505 = while {
    tunnel: w22 -> [_]
    tunnel: w18 -> [_]
    stop <- w1047 stop-if-true
    w1032 = 0.05 ("Sampling Time dt (s)")
    # "If dT and deadtime have similar values, the identification could evaluate deadtime as zero and this generates proportional gain equal to Inf. This code avoid gain changes in this situations."
    # "Autotuning Loop"
    n506 = local read "Control Output 12"() -> (w1049:dbl[])
    n507 = local read "Measurement 12"() -> (w1048:dbl[])
    n508 = Multiply(x=w1032, y=1000.0) -> (x*y=w1034:dbl)
    n509 = Wait Until Next ms Multiple(millisecond multiple=w1034) -> ()  [unwired: 1 out]
    n510 = case shown="\"Ziegler-Nichols\", Default" "Control 12" {
      tunnel: w1049 -> [w1058 w1066 w1075 w1084]
      tunnel: w1048 -> [w1057 w1065 w1074 w1083]
      tunnel: [w1056 w1064 w1073 w1082] -> w1036
      tunnel: [w1055 w1063 w1072 w1081] -> w1037
      tunnel: w1032 -> [w1054 w1062 w1071 w1080]
      tunnel: [w1053 w1061 w1070 w1079] -> w1035
      tunnel: [w1052 w1060 w1069 w1078] -> w1039
      tunnel: "Type of controller 12" -> [w1051 w1059 w1068 w1077]
      frame "Ziegler-Nichols", Default {
        n511 = call-poly <vilib>:"PID Autotuning Design.vi"("Ziegler-Nichols Speed"="Ziegler-Nichols speed 12", "Type of Controller"=w1051, "dt (s)"=w1054, "Response signal"=w1057, "Stimulus signal"=w1058) -> ("PID gains"=w1052:T3, "response operating point"=w1055:dbl, "stimulus operating point"=w1056:dbl, "Plant Parameters"=w1053:T5)  [unwired: 3 in]
      }
      frame "Cohen-Coon" {
        n512 = call-poly <vilib>:"PID Autotuning Design.vi"("Type of Controller"=w1059, "dt (s)"=w1062, "Response signal"=w1065, "Stimulus signal"=w1066) -> ("PID gains"=w1060:T3, "response offset"=w1063:dbl, "stimulus offset"=w1064:dbl, "Plant Parameters"=w1061:T5)  [unwired: 4 in]
      }
      frame "Chien-Hrones-Reswick" {
        n513 = call-poly <vilib>:"PID Autotuning Design.vi"("Tuning specifications"="Tuning specifications 12", "Type of Controller"=w1068, "dt (s)"=w1071, "Response signal"=w1074, "Stimulus signal"=w1075) -> ("PID gains"=w1069:T3, "response offset"=w1072:dbl, "stimulus offset"=w1073:dbl, "Plant Parameters"=w1070:T5)  [unwired: 3 in]
      }
      frame "Internal Model Control" {
        n514 = call-poly <vilib>:"PID Autotuning Design.vi"("Desired Time Constant (tau_c)"="Multiplicative factor 12", "Type of Controller"=w1077, "dt (s)"=w1080, "Response signal"=w1083, "Stimulus signal"=w1084) -> ("PID gains"=w1078:T3, "response offset"=w1081:dbl, "stimulus offset"=w1082:dbl, "Plant Parameters"=w1079:T5)  [unwired: 3 in]
      }
    }
    "Identified Plant Parameters 12" <- w1035
    "Response operating point 12" <- w1037
    "Stimulus operating point 12" <- w1036
    n515 = Unbundle(w1039) -> ("proportional gain (Kc)"=w1042:dbl)  [unwired: 2 out]
    n516 = Equal?(x=w1042, y=inf) -> (x = y?=w1041:bool)
    n517 = feedback #16() -> (w1040:T3)  [unwired: 1 in]
    n518 = Select(t=w1040, s=w1041, f=w1039) -> (s? t:f=w1038:T3)
    "Tuned PID gains 12" <- w1038
    n519 = feedback-in #16(w1038) -> ()
    n520 = case shown="True" "Accept gain 12" {
      tunnel: w1038 -> [_ w1085]
      frame False {
      }
      frame True {
        n521 = local write "PID Gains 12"(w1085) -> ()
      }
    }
    n522 = local read "Stop 12"() -> (w1047:bool)
  }
  n523 = while {
    tunnel: w34 -> [_]
    tunnel: w30 -> [_]
    stop <- w1101 stop-if-true
    w1086 = 0.05 ("Sampling Time dt (s)")
    # "If dT and deadtime have similar values, the identification could evaluate deadtime as zero and this generates proportional gain equal to Inf. This code avoid gain changes in this situations."
    # "Autotuning Loop"
    n524 = local read "Control Output 8"() -> (w1103:dbl[])
    n525 = local read "Measurement 8"() -> (w1102:dbl[])
    n526 = Multiply(x=w1086, y=1000.0) -> (x*y=w1088:dbl)
    n527 = Wait Until Next ms Multiple(millisecond multiple=w1088) -> ()  [unwired: 1 out]
    n528 = case shown="\"Chien-Hrones-Reswick\"" "Control 8" {
      tunnel: w1103 -> [w1112 w1120 w1129 w1138]
      tunnel: w1102 -> [w1111 w1119 w1128 w1137]
      tunnel: [w1110 w1118 w1127 w1136] -> w1091
      tunnel: [w1109 w1117 w1126 w1135] -> w1090
      tunnel: w1086 -> [w1108 w1116 w1125 w1134]
      tunnel: [w1107 w1115 w1124 w1133] -> w1089
      tunnel: [w1106 w1114 w1123 w1132] -> w1093
      tunnel: "Type of controller 8" -> [w1105 w1113 w1122 w1131]
      frame "Ziegler-Nichols", Default {
        n529 = call-poly <vilib>:"PID Autotuning Design.vi"("Ziegler-Nichols Speed"="Ziegler-Nichols speed 8", "Type of Controller"=w1105, "dt (s)"=w1108, "Response signal"=w1111, "Stimulus signal"=w1112) -> ("PID gains"=w1106:T3, "response operating point"=w1109:dbl, "stimulus operating point"=w1110:dbl, "Plant Parameters"=w1107:T5)  [unwired: 3 in]
      }
      frame "Cohen-Coon" {
        n530 = call-poly <vilib>:"PID Autotuning Design.vi"("Type of Controller"=w1113, "dt (s)"=w1116, "Response signal"=w1119, "Stimulus signal"=w1120) -> ("PID gains"=w1114:T3, "response offset"=w1117:dbl, "stimulus offset"=w1118:dbl, "Plant Parameters"=w1115:T5)  [unwired: 4 in]
      }
      frame "Chien-Hrones-Reswick" {
        n531 = call-poly <vilib>:"PID Autotuning Design.vi"("Tuning specifications"="Tuning specifications 8", "Type of Controller"=w1122, "dt (s)"=w1125, "Response signal"=w1128, "Stimulus signal"=w1129) -> ("PID gains"=w1123:T3, "response offset"=w1126:dbl, "stimulus offset"=w1127:dbl, "Plant Parameters"=w1124:T5)  [unwired: 3 in]
      }
      frame "Internal Model Control" {
        n532 = call-poly <vilib>:"PID Autotuning Design.vi"("Desired Time Constant (tau_c)"="Multiplicative factor 8", "Type of Controller"=w1131, "dt (s)"=w1134, "Response signal"=w1137, "Stimulus signal"=w1138) -> ("PID gains"=w1132:T3, "response offset"=w1135:dbl, "stimulus offset"=w1136:dbl, "Plant Parameters"=w1133:T5)  [unwired: 3 in]
      }
    }
    "Stimulus operating point 8" <- w1091
    "Response operating point 8" <- w1090
    "Identified Plant Parameters 8" <- w1089
    n533 = Unbundle(w1093) -> ("proportional gain (Kc)"=w1096:dbl)  [unwired: 2 out]
    n534 = Equal?(x=w1096, y=inf) -> (x = y?=w1095:bool)
    n535 = feedback #17() -> (w1094:T3)  [unwired: 1 in]
    n536 = Select(t=w1094, s=w1095, f=w1093) -> (s? t:f=w1092:T3)
    "Tuned PID gains 8" <- w1092
    n537 = feedback-in #17(w1092) -> ()
    n538 = case shown="True" "Accept gain 8" {
      tunnel: w1092 -> [_ w1139]
      frame False {
      }
      frame True {
        n539 = local write "PID Gains 8"(w1139) -> ()
      }
    }
    n540 = local read "Stop 8"() -> (w1101:bool)
  }
  n541 = while {
    stop <- w1155 stop-if-true
    w1140 = 0.05 ("Sampling Time dt (s)")
    # "If dT and deadtime have similar values, the identification could evaluate deadtime as zero and this generates proportional gain equal to Inf. This code avoid gain changes in this situations."
    # "Autotuning Loop"
    n542 = local read "Control Output 7"() -> (w1157:dbl[])
    n543 = local read "Measurement 7"() -> (w1156:dbl[])
    n544 = Multiply(x=w1140, y=1000.0) -> (x*y=w1142:dbl)
    n545 = Wait Until Next ms Multiple(millisecond multiple=w1142) -> ()  [unwired: 1 out]
    n546 = case shown="\"Chien-Hrones-Reswick\"" "Control 7" {
      tunnel: w1157 -> [w1166 w1174 w1183 w1192]
      tunnel: w1156 -> [w1165 w1173 w1182 w1191]
      tunnel: [w1164 w1172 w1181 w1190] -> w1145
      tunnel: [w1163 w1171 w1180 w1189] -> w1144
      tunnel: w1140 -> [w1162 w1170 w1179 w1188]
      tunnel: [w1161 w1169 w1178 w1187] -> w1143
      tunnel: [w1160 w1168 w1177 w1186] -> w1147
      tunnel: "Type of controller 7" -> [w1159 w1167 w1176 w1185]
      frame "Ziegler-Nichols", Default {
        n547 = call-poly <vilib>:"PID Autotuning Design.vi"("Ziegler-Nichols Speed"="Ziegler-Nichols speed 7", "Type of Controller"=w1159, "dt (s)"=w1162, "Response signal"=w1165, "Stimulus signal"=w1166) -> ("PID gains"=w1160:T3, "response operating point"=w1163:dbl, "stimulus operating point"=w1164:dbl, "Plant Parameters"=w1161:T5)  [unwired: 3 in]
      }
      frame "Cohen-Coon" {
        n548 = call-poly <vilib>:"PID Autotuning Design.vi"("Type of Controller"=w1167, "dt (s)"=w1170, "Response signal"=w1173, "Stimulus signal"=w1174) -> ("PID gains"=w1168:T3, "response offset"=w1171:dbl, "stimulus offset"=w1172:dbl, "Plant Parameters"=w1169:T5)  [unwired: 4 in]
      }
      frame "Chien-Hrones-Reswick" {
        n549 = call-poly <vilib>:"PID Autotuning Design.vi"("Tuning specifications"="Tuning specifications 7", "Type of Controller"=w1176, "dt (s)"=w1179, "Response signal"=w1182, "Stimulus signal"=w1183) -> ("PID gains"=w1177:T3, "response offset"=w1180:dbl, "stimulus offset"=w1181:dbl, "Plant Parameters"=w1178:T5)  [unwired: 3 in]
      }
      frame "Internal Model Control" {
        n550 = call-poly <vilib>:"PID Autotuning Design.vi"("Desired Time Constant (tau_c)"="Multiplicative factor 7", "Type of Controller"=w1185, "dt (s)"=w1188, "Response signal"=w1191, "Stimulus signal"=w1192) -> ("PID gains"=w1186:T3, "response offset"=w1189:dbl, "stimulus offset"=w1190:dbl, "Plant Parameters"=w1187:T5)  [unwired: 3 in]
      }
    }
    "Stimulus operating point 7" <- w1145
    "Response operating point 7" <- w1144
    "Identified Plant Parameters 7" <- w1143
    n551 = Unbundle(w1147) -> ("proportional gain (Kc)"=w1150:dbl)  [unwired: 2 out]
    n552 = Equal?(x=w1150, y=inf) -> (x = y?=w1149:bool)
    n553 = feedback #18() -> (w1148:T3)  [unwired: 1 in]
    n554 = Select(t=w1148, s=w1149, f=w1147) -> (s? t:f=w1146:T3)
    "Tuned PID gains 7" <- w1146
    n555 = feedback-in #18(w1146) -> ()
    n556 = case shown="True" "Accept gain 7" {
      tunnel: w1146 -> [_ w1193]
      frame False {
      }
      frame True {
        n557 = local write "PID Gains 7"(w1193) -> ()
      }
    }
    n558 = local read "Stop 7"() -> (w1155:bool)
  }
  n559 = call <instrlib>:"PDI close.vi"("error in (no error)"=w64, "pDev"=w70) -> ("error out"=→"error out":errorcluster, "connected"=w65:bool)  [unwired: 8 out]
  n560 = local write "Connected"(w65) -> ()
